vi "Parse Uplink.vi"(8 "error in (no error)":errorcluster, 10 "Uplink":u8[][](array[numeric]) format="%02x") -> (0 "error out":errorcluster, 1 "Data":string, 2 "Response Code":string, 3 "Response Token":string, 4 "tChecksum Valid":bool, 5 "CP_DATA":u8[](array[numeric]), 6 "bChecksum Valid":bool)   [LabVIEW 2009]
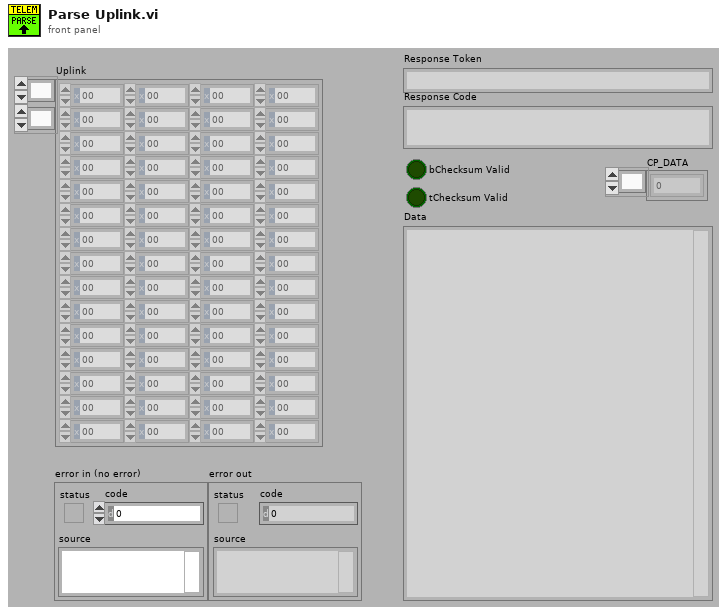
[diagram p1: front panel]
types:
  T1 = cluster{"FirstBlockFlag":u8, "respToken":u8, "cmdToken":u16, "cmdData":u8[], "b1ChkSum":u8, "tChkSum":u8, "tChkSumCalc":u8, "b1ChkSumCalc":u8}
  T2 = cluster{"Boolean array[0]":bool, "Boolean array[1]":bool, "Boolean array[2]":bool, "Boolean array[3]":bool, "Boolean array[4]":bool, "Boolean array[5]":bool, "Boolean array[6]":bool, "Boolean array[7]":bool}
  T3 = cluster{"Boolean array[0]":bool, "Boolean array[1]":bool, "Boolean array[2]":bool, "Boolean array[3]":bool, "Boolean array[4]":bool, "Boolean array[5]":bool, "Boolean array[6]":bool, "Boolean array[7]":bool, "Boolean array[8]":bool, "Boolean array[9]":bool, "Boolean array[10]":bool, "Boolean array[11]":bool, "Boolean array[12]":bool, "Boolean array[13]":bool, "Boolean array[14]":bool, "Boolean array[15]":bool}
  T4 = cluster{"DATA[0]":u8, "DATA[1]":u8, "DATA[2]":u8, "DATA[3]":u8, "DATA[4]":u8, "DATA[5]":u8, "DATA[6]":u8, "DATA[7]":u8}
  T5 = cluster{"[0]":string, "[1]":string, "[2]":string, "[3]":string, "[4]":string, "[5]":string, "[6]":string, "[7]":string, "[8]":string, "[9]":string}
  T6 = cluster{"DATA[0]":u8, "DATA[1]":u8, "DATA[2]":u8, "DATA[3]":u8, "DATA[4]":u8, "DATA[5]":u8, "DATA[6]":u8, "DATA[7]":u8, "DATA[8]":u8, "DATA[9]":u8, "DATA[10]":u8, "DATA[11]":u8, "DATA[12]":u8, "DATA[13]":u8, "DATA[14]":u8, "DATA[15]":u8}
  T7 = cluster{"[0]":u8, "[1]":u8, "[2]":u8, "[3]":u8, "[4]":u8, "[5]":u8, "[6]":u8, "[7]":u8, "[8]":u8, "[9]":u8, "[10]":u8, "[11]":u8, "[12]":u8, "[13]":u8, "[14]":u8, "[15]":u8, "[16]":u8, "[17]":u8, "[18]":u8, "[19]":u8, "[20]":u8, "[21]":u8, "[22]":u8, "[23]":u8, "[24]":u8, "[25]":u8, "[26]":u8, "[27]":u8, "[28]":u8, "[29]":u8, "[30]":u8, "[31]":u8, "[32]":u8, "[33]":u8, "[34]":u8, "[35]":u8, "[36]":u8, "[37]":u8, "[38]":u8, "[39]":u8, "[40]":u8, "[41]":u8, "[42]":u8, "[43]":u8, "[44]":u8, "[45]":u8, "[46]":u8, "[47]":u8, "[48]":u8, "[49]":u8, "[50]":u8, "[51]":u8, "[52]":u8, "[53]":u8}
  T8 = cluster{"DATA[0]":u8, "DATA[1]":u8, "DATA[2]":u8, "DATA[3]":u8, "DATA[4]":u8, "DATA[5]":u8, "DATA[6]":u8, "DATA[7]":u8, "DATA[8]":u8, "DATA[9]":u8, "DATA[10]":u8, "DATA[11]":u8, "DATA[12]":u8, "DATA[13]":u8, "DATA[14]":u8, "DATA[15]":u8, "DATA[16]":u8, "DATA[17]":u8, "DATA[18]":u8, "DATA[19]":u8, "DATA[20]":u8, "DATA[21]":u8, "DATA[22]":u8, "DATA[23]":u8, "DATA[24]":u8, "DATA[25]":u8, "DATA[26]":u8, "DATA[27]":u8, "DATA[28]":u8, "DATA[29]":u8, "DATA[30]":u8, "DATA[31]":u8, "DATA[32]":u8, "DATA[33]":u8, "DATA[34]":u8, "DATA[35]":u8, "DATA[36]":u8, "DATA[37]":u8, "DATA[38]":u8, "DATA[39]":u8, "DATA[40]":u8, "DATA[41]":u8, "DATA[42]":u8, "DATA[43]":u8, "DATA[44]":u8, "DATA[45]":u8, "DATA[46]":u8}
  T9 = cluster{"DATA[0]":u8, "DATA[1]":u8, "DATA[2]":u8, "DATA[3]":u8, "DATA[4]":u8, "DATA[5]":u8, "DATA[6]":u8, "DATA[7]":u8, "DATA[8]":u8, "DATA[9]":u8, "DATA[10]":u8, "DATA[11]":u8, "DATA[12]":u8, "DATA[13]":u8, "DATA[14]":u8, "DATA[15]":u8, "DATA[16]":u8, "DATA[17]":u8, "DATA[18]":u8, "DATA[19]":u8, "DATA[20]":u8, "DATA[21]":u8, "DATA[22]":u8, "DATA[23]":u8}
  T10 = cluster{"Boolean array[0]":bool, "Boolean array[1]":bool, "Boolean array[2]":bool, "Boolean array[3]":bool, "Boolean array[4]":bool, "Boolean array[5]":bool, "Boolean array[6]":bool, "Boolean array[7]":bool, "Boolean array[8]":bool}
  T11 = cluster{"[0]":u8, "[1]":u8, "[2]":u8, "[3]":u8, "[4]":u8, "[5]":u8, "[6]":u8, "[7]":u8}
  T12 = cluster{"[0]":u8, "[1]":u8, "[2]":u8, "[3]":u8, "[4]":u8, "[5]":u8, "[6]":u8, "[7]":u8, "[8]":u8, "[9]":u8, "[10]":u8, "[11]":u8, "[12]":u8, "[13]":u8, "[14]":u8, "[15]":u8, "[16]":u8, "[17]":u8, "[18]":u8, "[19]":u8, "[20]":u8, "[21]":u8, "[22]":u8, "[23]":u8, "[24]":u8, "[25]":u8, "[26]":u8, "[27]":u8, "[28]":u8, "[29]":u8, "[30]":u8, "[31]":u8, "[32]":u8, "[33]":u8, "[34]":u8, "[35]":u8, "[36]":u8, "[37]":u8}
  T13 = cluster{"[0]":u8, "[1]":u8, "[2]":u8, "[3]":u8, "[4]":u8, "[5]":u8}
  T14 = cluster{"DATA[0]":u8, "DATA[1]":u8, "DATA[2]":u8, "DATA[3]":u8, "DATA[4]":u8, "DATA[5]":u8}
  T15 = cluster{"DATA[0]":u8, "DATA[1]":u8, "DATA[2]":u8, "DATA[3]":u8, "DATA[4]":u8, "DATA[5]":u8, "DATA[6]":u8, "DATA[7]":u8, "DATA[8]":u8, "DATA[9]":u8, "DATA[10]":u8, "DATA[11]":u8, "DATA[12]":u8, "DATA[13]":u8, "DATA[14]":u8, "DATA[15]":u8, "DATA[16]":u8}
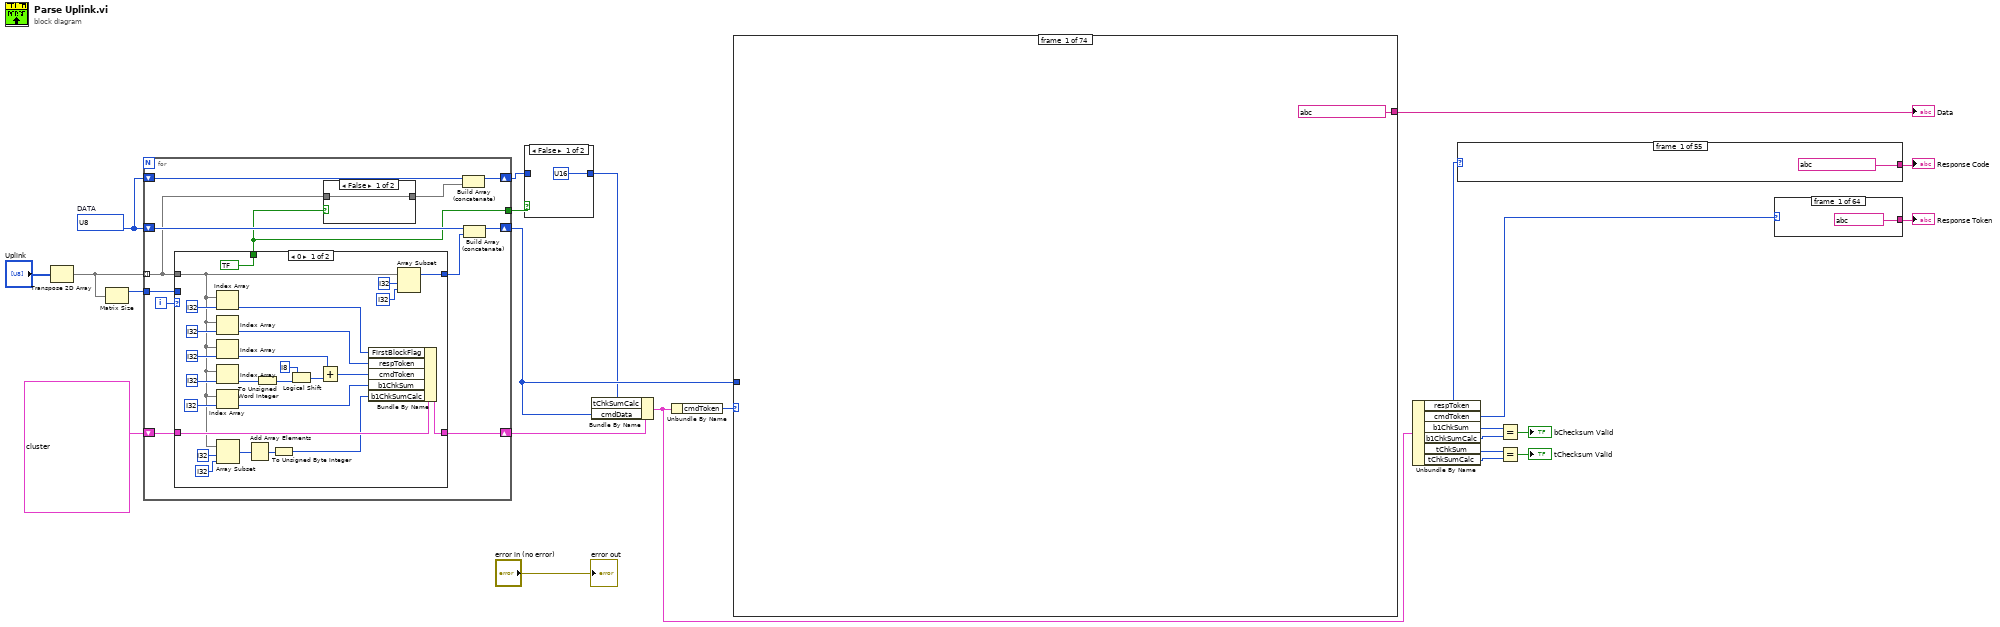
[diagram p0: block diagram]
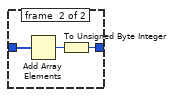
[diagram p2: hidden frame]
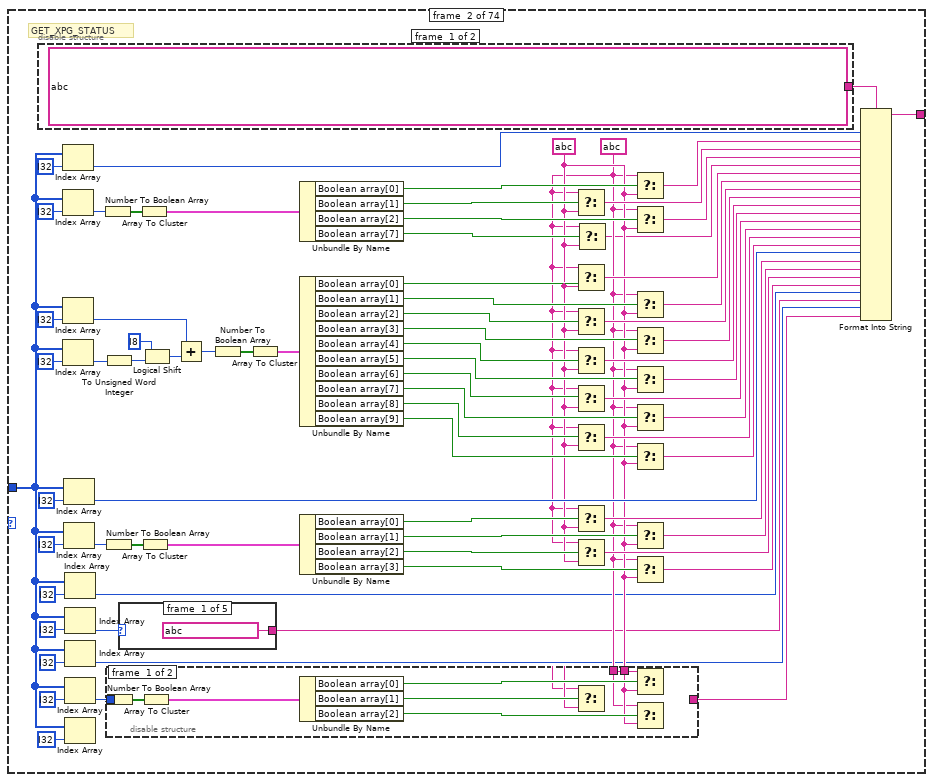
[diagram p3: hidden frame]
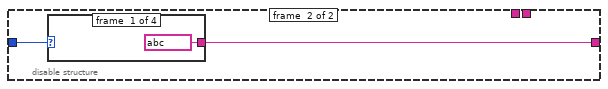
[diagram p4: hidden frame]
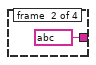
[diagram p5: hidden frame]
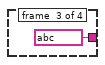
[diagram p6: hidden frame]
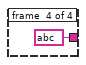
[diagram p7: hidden frame]
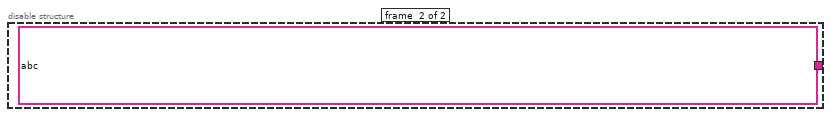
[diagram p8: hidden frame]
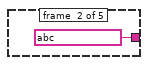
[diagram p9: hidden frame]
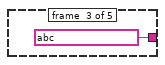
[diagram p10: hidden frame]
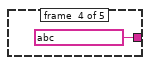
[diagram p11: hidden frame]
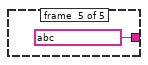
[diagram p12: hidden frame]
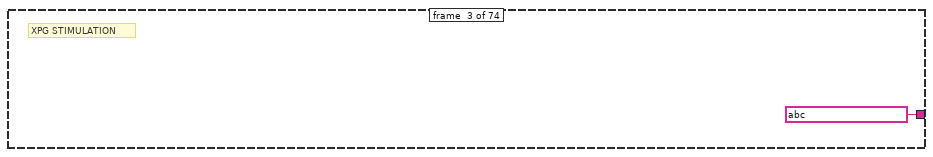
[diagram p13: hidden frame]
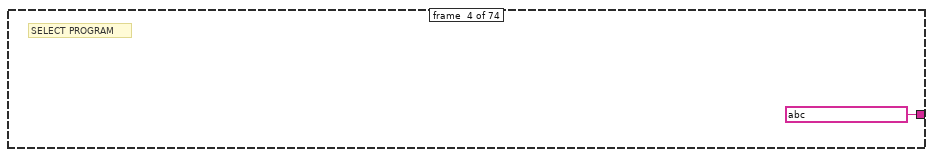
[diagram p14: hidden frame]
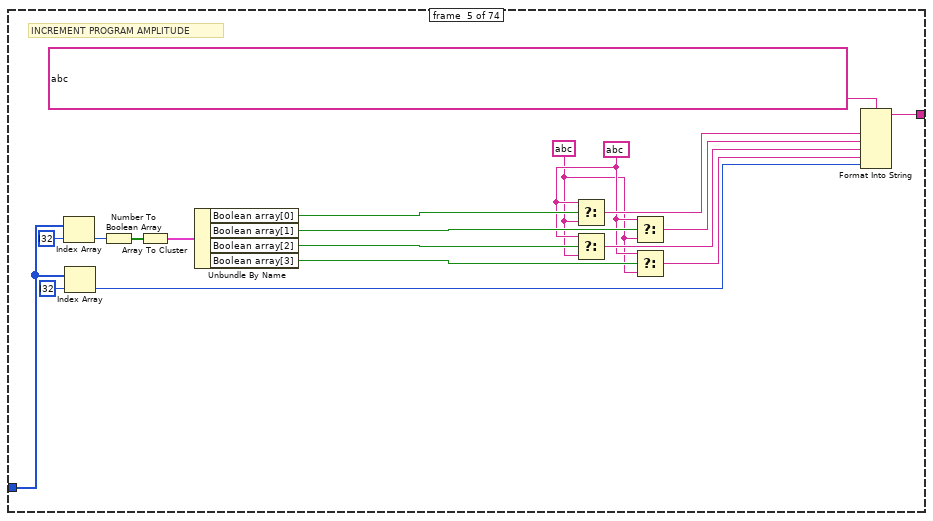
[diagram p15: hidden frame]
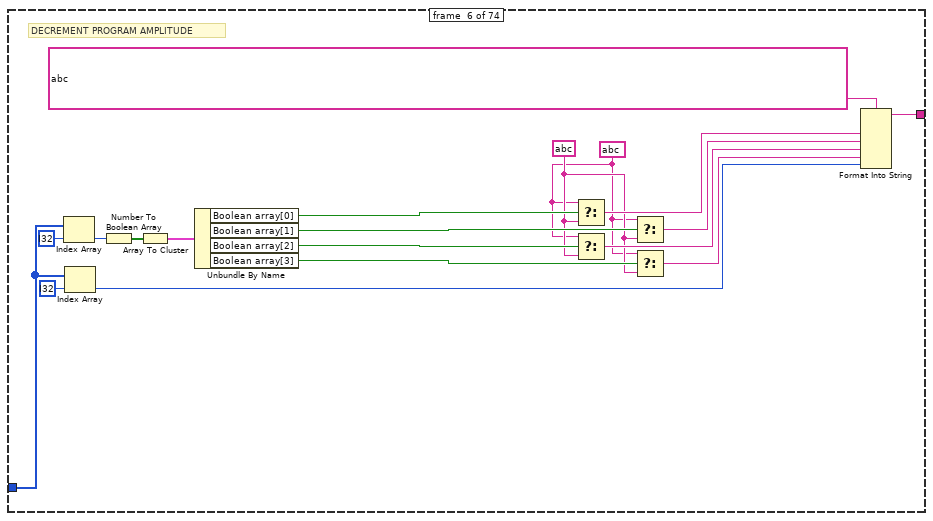
[diagram p16: hidden frame]
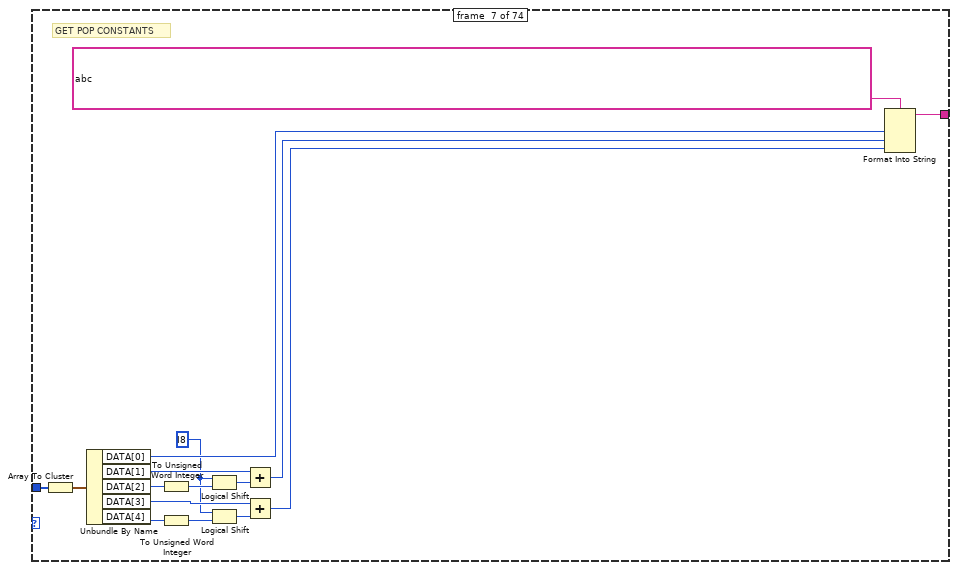
[diagram p17: hidden frame]
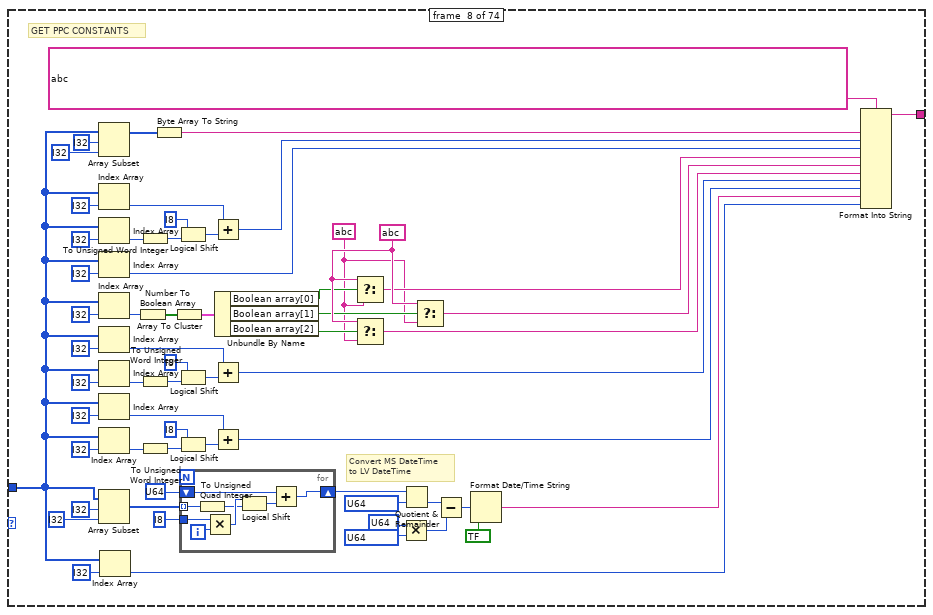
[diagram p18: hidden frame]
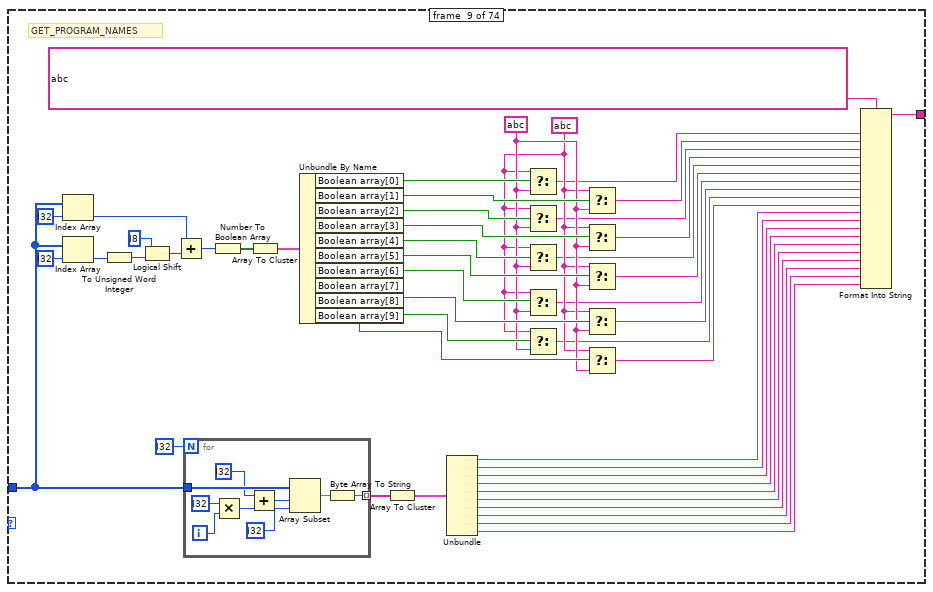
[diagram p19: hidden frame]
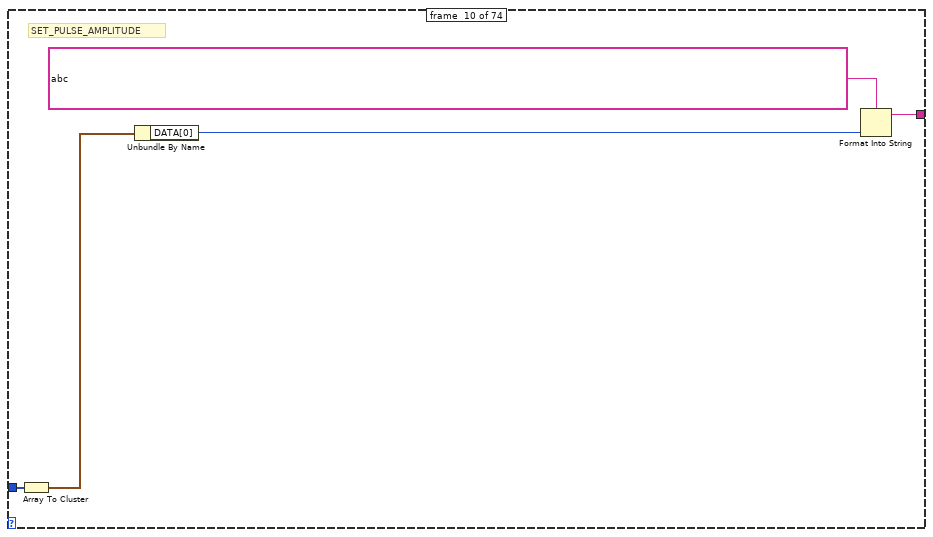
[diagram p20: hidden frame]
diagram:
  w13 = u8[] ?  # DATA
  n1 = Transpose 2D Array(2D array="Uplink") -> (transposed array=w15:u8[][])
  n2 = Matrix Size(0:w15) -> (1:w21:i32)  [unwired: 1 out]
  n3 = for {
    tunnel: w15 -> [w27] mode=indexing
    shift-right: [w31] -> w19
    shift-left: w13 -> [w32]
    shift-right: [w34] -> w20
    shift-left: T1 ? -> [w35]
    tunnel: w21 -> [w33]
    shift-right: [w28] -> w12
    shift-left: w13 -> [w29]
    tunnel: [w25] -> w11
    i -> [w36]
    n4 = case shown="0" w36 {
      selector: w36 -> [_ w79]
      tunnel: w27 -> [w45 w69]
      tunnel: [w65 w75] -> w30
      tunnel: w35 -> [w59 w70]
      tunnel: [w58 w71] -> w34
      tunnel: w33 -> [_ w77]
      tunnel: [bool ? w68] -> w25
      frame #0 {
        n5 = Index Array(array=w45, index=i32 ?) -> (element=w57:u8)
        n6 = Index Array(array=w45, index=i32 ?) -> (element=w54:u8)
        n7 = Index Array(array=w45, index=i32 ?) -> (element=w49:u8)
        n8 = Index Array(array=w45, index=i32 ?) -> (element=w53:u8)
        n9 = Index Array(array=w45, index=i32 ?) -> (element=w56:u8)
        n10 = Array Subset(array=w45, index=i32 ?, length=i32 ?) -> (w42:u8[])
        n11 = Add Array Elements(numeric array=w42) -> (sum=w44:u8)
        n12 = To Unsigned Word Integer(number=w53) -> (unsigned 16bit integer=w55:u16)
        n13 = To Unsigned Byte Integer(number=w44) -> (unsigned 8bit integer=w43:u8)
        n14 = Logical Shift(y=i8 ?, x=w55) -> (x << y=w51:u16)
        n15 = Add(x=w49, y=w51) -> (x+y=w50:u16)
        n16 = Bundle By Name(cluster=w59, "FirstBlockFlag"=w57, "respToken"=w54, "cmdToken"=w50, "b1ChkSum"=w56, "b1ChkSumCalc"=w43) -> (w58:T1)
        n17 = Array Subset(array=w45, index=i32 ?, length=i32 ?) -> (w65:u8[])
      }
      frame #1 {
        # "If Last Packet of Multi-Packet\nUplink, truncate Data Read\nand store tChkSum"
        n18 = Increment(x=w79) -> (x+1=w78:i32)
        n19 = Equal?(x=w77, y=w78) -> (x = y?=w68:bool)
        n20 = case shown="True" w68 {
          tunnel: [w80 w84] -> w71
          tunnel: w70 -> [w80 w85]
          tunnel: w69 -> [_ w82]
          frame #0 {
          }
          frame #1 {
            n21 = Index Array(array=w82, index=i32 ?) -> (element=w83:u8)
            n22 = Bundle By Name(cluster=w85, "tChkSum"=w83) -> (w84:T1)
          }
        }
        n23 = Select(t=i32 ? ("length"), s=w68, f=i32 ? ("length")) -> (s? t:f=w74:i32)
        n24 = Array Subset(array=w69, index=i32 ?, length=w74) -> (w75:u8[])
      }
    }
    n25 = case shown="False" w25 {
      tunnel: w27 -> [w37 w40]
      tunnel: [w37 w39] -> w26
      frame #0 {
      }
      frame #1 {
        n26 = Array Subset(array=w40, index=i32 ?, length=i32 ?) -> (w39:u8[])
      }
    }
    n27 = Build Array (concatenate)(w29, w26) -> (w28:u8[])
    n28 = Build Array (concatenate)(w32, w30) -> (w31:u8[])
  }
  n29 = case shown="False" w11 {
    tunnel: w12 -> [_ w87]
    tunnel: [u16 ? ("CRC16r") w88] -> w2
    frame #0 {
    }
    frame #1 {
      n30 = Add Array Elements(numeric array=w87) -> (sum=w89:u8)
      n31 = To Unsigned Byte Integer(number=w89) -> (unsigned 8bit integer=w88:u8)
    }
  }
  n32 = Bundle By Name(cluster=w20, "tChkSumCalc"=w2, "cmdData"=w19) -> (w4:T1)
  n33 = Unbundle By Name(w4) -> ("cmdToken"=w1:u16)
  n34 = case shown="3" w1 {
    tunnel: w19 -> [_ w100 _ _ w194 w213 w232 w241 w323 w369 w374 w379 w395 _ w414 w419 w424 _ w430 w435 w450 w469 _ _ w478 _ w615 _ w648 _ w798 _ w807 _ w855 _ w902 _ w928 _ w954 w962 w998 w1020 _ w1028 _ w1053 w1058 w1073 _ w1166 _ w1191 _ w1200 _ w1260 _ w1316 _ w1321 _ _ _ w1335 _ _ _ _ w1363 _ w1431 _]
    tunnel: [string ? w162 string ? string ? w204 w223 w239 w300 w356 w370 w375 w380 w409 string ? w415 w420 w425 string ? w431 w436 w451 w473 string ? string ? w517 string ? w626 string ? w713 string ? w802 string ? w812 string ? w860 string ? w905 string ? w931 string ? w956 w973 w1000 w1022 string ? w1033 string ? w1055 w1062 w1104 string ? w1169 string ? w1196 string ? w1208 string ? w1267 string ? w1317 string ? w1329 _ _ string ? w1343 _ _ _ _ w1366 string ? w1433 string ?] -> w18
    frame #0 {
    }
    frame #1 {
      w98 = string ?
      w97 = string ?
      # "GET_XPG_STATUS"
      n35 = disable-structure shown="Enabled" {
        disable-tunnel: [_ string ? ("format string")] -> w91
        frame #0 {
          (unwired) string ? ("format string")
        }
        frame #1 {
        }
      }
      n36 = Index Array(array=w100, index=i32 ?) -> (element=w163:u8)
      n37 = Index Array(array=w100, index=i32 ?) -> (element=w147:u8)
      n38 = Index Array(array=w100, index=i32 ?) -> (element=w135:u8)
      n39 = Index Array(array=w100, index=i32 ?) -> (element=w136:u8)
      n40 = Index Array(array=w100, index=i32 ?) -> (element=w120:u8)
      n41 = Index Array(array=w100, index=i32 ?) -> (element=w118:u8)
      n42 = Index Array(array=w100, index=i32 ?) -> (element=w95:u8)
      n43 = Index Array(array=w100, index=i32 ?) -> (element=w105:u8)
      n44 = Index Array(array=w100, index=i32 ?) -> (element=w93:u8)
      n45 = Index Array(array=w100, index=i32 ?) -> (element=w102:u8)
      n46 = Index Array(array=w100, index=i32 ?) -> ()  [unwired: 1 out]
      n47 = Number To Boolean Array(number=w147) -> (Boolean array=w146:bool[])
      n48 = To Unsigned Word Integer(number=w136) -> (unsigned 16bit integer=w139:u16)
      n49 = Number To Boolean Array(number=w118) -> (Boolean array=w117:bool[])
      n50 = disable-structure shown="Enabled" {
        disable-tunnel: w102 -> [w172 w174]
        disable-tunnel: w98 -> [w166 _]
        disable-tunnel: w97 -> [w165 _]
        disable-tunnel: [_ w173] -> w92
        frame #0 {
          n51 = Number To Boolean Array(number=w172) -> (Boolean array=w171:bool[])
          n52 = Array To Cluster(array=w171) -> (cluster=w170:T2)
          n53 = Unbundle By Name(w170) -> ("Boolean array[0]"=w169:bool, "Boolean array[1]"=w168:bool, "Boolean array[2]"=w167:bool)
          n54 = Select(t=w165, s=w168, f=w166) -> ()  [unwired: 1 out]
          n55 = Select(t=w165, s=w169, f=w166) -> ()  [unwired: 1 out]
          n56 = Select(t=w165, s=w167, f=w166) -> ()  [unwired: 1 out]
        }
        frame #1 {
          n57 = case shown="3" w174 {
            tunnel: [string ? string ? string ? string ?] -> w173
            frame #0 {
            }
            frame #1 {
            }
            frame #2 {
            }
            frame #3 {
            }
          }
        }
      }
      n58 = case shown="4" w105 {
        tunnel: [string ? string ? string ? string ? string ?] -> w94
        frame #0 {
        }
        frame #1 {
        }
        frame #2 {
        }
        frame #3 {
        }
        frame #4 {
        }
      }
      n59 = Array To Cluster(array=w146) -> (cluster=w145:T2)
      n60 = Array To Cluster(array=w117) -> (cluster=w116:T2)
      n61 = Logical Shift(y=i8 ?, x=w139) -> (x << y=w137:u16)
      n62 = Add(x=w135, y=w137) -> (x+y=w133:u16)
      n63 = Number To Boolean Array(number=w133) -> (Boolean array=w134:bool[])
      n64 = Array To Cluster(array=w134) -> (cluster=w132:T3)
      n65 = Unbundle By Name(w145) -> ("Boolean array[0]"=w144:bool, "Boolean array[1]"=w143:bool, "Boolean array[2]"=w142:bool, "Boolean array[7]"=w99:bool)
      n66 = Unbundle By Name(w132) -> ("Boolean array[0]"=w131:bool, "Boolean array[1]"=w130:bool, "Boolean array[2]"=w129:bool, "Boolean array[3]"=w128:bool, "Boolean array[4]"=w127:bool, "Boolean array[5]"=w126:bool, "Boolean array[6]"=w125:bool, "Boolean array[7]"=w124:bool, "Boolean array[8]"=w123:bool, "Boolean array[9]"=w122:bool)
      n67 = Unbundle By Name(w116) -> ("Boolean array[0]"=w115:bool, "Boolean array[1]"=w114:bool, "Boolean array[2]"=w113:bool, "Boolean array[3]"=w112:bool)
      n68 = Select(t=w97, s=w143, f=w98) -> (s? t:f=w160:string)
      n69 = Select(t=w97, s=w131, f=w98) -> (s? t:f=w158:string)
      n70 = Select(t=w97, s=w129, f=w98) -> (s? t:f=w156:string)
      n71 = Select(t=w97, s=w127, f=w98) -> (s? t:f=w154:string)
      n72 = Select(t=w97, s=w125, f=w98) -> (s? t:f=w152:string)
      n73 = Select(t=w97, s=w123, f=w98) -> (s? t:f=w150:string)
      n74 = Select(t=w97, s=w115, f=w98) -> (s? t:f=w111:string)
      n75 = Select(t=w97, s=w113, f=w98) -> (s? t:f=w109:string)
      n76 = Select(t=w97, s=w99, f=w98) -> (s? t:f=w96:string)
      n77 = Select(t=w97, s=w144, f=w98) -> (s? t:f=w161:string)
      n78 = Select(t=w97, s=w142, f=w98) -> (s? t:f=w159:string)
      n79 = Select(t=w97, s=w130, f=w98) -> (s? t:f=w157:string)
      n80 = Select(t=w97, s=w128, f=w98) -> (s? t:f=w155:string)
      n81 = Select(t=w97, s=w126, f=w98) -> (s? t:f=w153:string)
      n82 = Select(t=w97, s=w124, f=w98) -> (s? t:f=w151:string)
      n83 = Select(t=w97, s=w122, f=w98) -> (s? t:f=w149:string)
      n84 = Select(t=w97, s=w114, f=w98) -> (s? t:f=w110:string)
      n85 = Select(t=w97, s=w112, f=w98) -> (s? t:f=w108:string)
      n86 = Format Into String(format string=w91, w163, w161, w160, w159, w96, w158, w157, w156, w155, w154, w153, w152, w151, w150, w149, w120, w111, w110, w109, w108, w95, w94, w93, w92) -> (resulting string=w162:string)  [unwired: 2 in, 1 out]
    }
    frame #2 {
      # "XPG STIMULATION"
    }
    frame #3 {
      # "SELECT PROGRAM"
    }
    frame #4 {
      w187 = string ?
      w188 = string ?
      # "INCREMENT PROGRAM AMPLITUDE"
      n87 = Index Array(array=w194, index=i32 ?) -> (element=w202:u8)
      n88 = Index Array(array=w194, index=i32 ?) -> (element=w189:u8)
      n89 = Number To Boolean Array(number=w202) -> (Boolean array=w201:bool[])
      n90 = Array To Cluster(array=w201) -> (cluster=w200:T2)
      n91 = Unbundle By Name(w200) -> ("Boolean array[0]"=w199:bool, "Boolean array[1]"=w198:bool, "Boolean array[2]"=w197:bool, "Boolean array[3]"=w196:bool)
      n92 = Select(t=w188, s=w199, f=w187) -> (s? t:f=w193:string)
      n93 = Select(t=w188, s=w197, f=w187) -> (s? t:f=w191:string)
      n94 = Select(t=w188, s=w198, f=w187) -> (s? t:f=w192:string)
      n95 = Select(t=w188, s=w196, f=w187) -> (s? t:f=w190:string)
      n96 = Format Into String(format string=string ?, w193, w192, w191, w190, w189) -> (resulting string=w204:string)  [unwired: 2 in, 1 out]
    }
    frame #5 {
      w207 = string ?
      w206 = string ?
      # "DECREMENT PROGRAM AMPLITUDE"
      n97 = Index Array(array=w213, index=i32 ?) -> (element=w221:u8)
      n98 = Index Array(array=w213, index=i32 ?) -> (element=w208:u8)
      n99 = Number To Boolean Array(number=w221) -> (Boolean array=w220:bool[])
      n100 = Array To Cluster(array=w220) -> (cluster=w219:T2)
      n101 = Unbundle By Name(w219) -> ("Boolean array[0]"=w218:bool, "Boolean array[1]"=w217:bool, "Boolean array[2]"=w216:bool, "Boolean array[3]"=w215:bool)
      n102 = Select(t=w206, s=w218, f=w207) -> (s? t:f=w212:string)
      n103 = Select(t=w206, s=w216, f=w207) -> (s? t:f=w210:string)
      n104 = Select(t=w206, s=w217, f=w207) -> (s? t:f=w211:string)
      n105 = Select(t=w206, s=w215, f=w207) -> (s? t:f=w209:string)
      n106 = Format Into String(format string=string ?, w212, w211, w210, w209, w208) -> (resulting string=w223:string)  [unwired: 2 in, 1 out]
    }
    frame #6 {
      w225 = i8 ? ("y")
      # "GET POP CONSTANTS"
      n107 = Array To Cluster(array=w232) -> (cluster=w231:T4)
      n108 = Unbundle By Name(w231) -> ("DATA[0]"=w230:u8, "DATA[1]"=w229:u8, "DATA[2]"=w228:u8, "DATA[3]"=w227:u8, "DATA[4]"=w226:u8)
      n109 = To Unsigned Word Integer(number=w228) -> (unsigned 16bit integer=w238:u16)
      n110 = To Unsigned Word Integer(number=w226) -> (unsigned 16bit integer=w236:u16)
      n111 = Logical Shift(y=w225, x=w238) -> (x << y=w237:u16)
      n112 = Logical Shift(y=w225, x=w236) -> (x << y=w235:u16)
      n113 = Add(x=w229, y=w237) -> (x+y=w234:u16)
      n114 = Add(x=w227, y=w235) -> (x+y=w233:u16)
      n115 = Format Into String(format string=string ?, w230, w234, w233) -> (resulting string=w239:string)  [unwired: 2 in, 1 out]
    }
    frame #7 {
      w243 = string ?
      w281 = string ?
      # "Convert MS DateTime\nto LV DateTime"
      # "GET PPC CONSTANTS"
      n116 = Array Subset(array=w241, index=i32 ?, length=i32 ?) -> (w297:u8[])
      n117 = Index Array(array=w241, index=i32 ?) -> (element=w289:u8)
      n118 = Index Array(array=w241, index=i32 ?) -> (element=w290:u8)
      n119 = Index Array(array=w241, index=i32 ?) -> (element=w286:u8)
      n120 = Index Array(array=w241, index=i32 ?) -> (element=w284:u8)
      n121 = Index Array(array=w241, index=i32 ?) -> (element=w268:u8)
      n122 = Index Array(array=w241, index=i32 ?) -> (element=w269:u8)
      n123 = Index Array(array=w241, index=i32 ?) -> (element=w260:u8)
      n124 = Index Array(array=w241, index=i32 ?) -> (element=w261:u8)
      n125 = Array Subset(array=w241, index=i32 ?, length=i32 ?) -> (w256:u8[])
      n126 = Index Array(array=w241, index=i32 ?) -> (element=w246:u8)
      n127 = Number To Boolean Array(number=w284) -> (Boolean array=w283:bool[])
      n128 = To Unsigned Word Integer(number=w290) -> (unsigned 16bit integer=w293:u16)
      n129 = To Unsigned Word Integer(number=w269) -> (unsigned 16bit integer=w272:u16)
      n130 = To Unsigned Word Integer(number=w261) -> (unsigned 16bit integer=w264:u16)
      n131 = Byte Array To String(unsigned byte array=w297) -> (string=w296:string)
      n132 = Array To Cluster(array=w283) -> (cluster=w282:T2)
      n133 = Logical Shift(y=i8 ?, x=w293) -> (x << y=w291:u16)
      n134 = Logical Shift(y=i8 ?, x=w272) -> (x << y=w270:u16)
      n135 = Logical Shift(y=i8 ?, x=w264) -> (x << y=w262:u16)
      n136 = for {
        tunnel: w256 -> [w309] mode=indexing
        shift-right: [w303] -> w251
        shift-left: u64 ? ("y") -> [w304]
        tunnel: i8 ? ("y") -> [w307]
        i -> [w308]
        n137 = To Unsigned Quad Integer(1:w309) -> (0:w302:u64)
        n138 = Multiply(x=w307, y=w308) -> (x*y=w306:i32)
        n139 = Logical Shift(y=w306, x=w302) -> (x << y=w305:u64)
        n140 = Add(x=w304, y=w305) -> (x+y=w303:u64)
      }
      n141 = Add(x=w289, y=w291) -> (x+y=w288:u16)
      n142 = Add(x=w268, y=w270) -> (x+y=w267:u16)
      n143 = Add(x=w260, y=w262) -> (x+y=w259:u16)
      n144 = Unbundle By Name(w282) -> ("Boolean array[0]"=w279:bool, "Boolean array[1]"=w280:bool, "Boolean array[2]"=w278:bool)
      n145 = Select(t=w281, s=w279, f=w243) -> (s? t:f=w277:string)
      n146 = Select(t=w281, s=w278, f=w243) -> (s? t:f=w275:string)
      n147 = Multiply(x=u64 ? ("y"), y=u64 ?) -> (x*y=w249:u64)
      n148 = Quotient & Remainder(x=w251, y=u64 ?) -> (floor(x/y)=w242:u64)  [unwired: 1 out]
      n149 = Select(t=w281, s=w280, f=w243) -> (s? t:f=w276:string)
      n150 = Subtract(x=w242, y=w249) -> (x-y=w245:u64)
      n151 = Format Date/Time String(seconds (now)=w245, UTC format=bool ?) -> (date/time string=w244:string)  [unwired: 1 in]
      n152 = Format Into String(format string=string ?, w296, w288, w286, w277, w276, w275, w267, w259, w244, w246) -> (resulting string=w300:string)  [unwired: 2 in, 1 out]
    }
    frame #8 {
      w335 = string ?
      w334 = string ?
      # "GET_PROGRAM_NAMES"
      n153 = Index Array(array=w323, index=i32 ?) -> (element=w349:u8)
      n154 = Index Array(array=w323, index=i32 ?) -> (element=w350:u8)
      n155 = To Unsigned Word Integer(number=w350) -> (unsigned 16bit integer=w353:u16)
      n156 = Logical Shift(y=i8 ?, x=w353) -> (x << y=w351:u16)
      n157 = Add(x=w349, y=w351) -> (x+y=w347:u16)
      n158 = for {
        N: i32 ? -> [_]
        tunnel: w323 -> [w366]
        tunnel: [w358] -> w322 mode=indexing
        i -> [w364]
        n159 = Multiply(x=i32 ?, y=w364) -> (x*y=w362:i32)
        n160 = Add(x=i32 ?, y=w362) -> (x+y=w360:i32)
        n161 = Array Subset(array=w366, index=w360, length=i32 ?) -> (w359:u8[])
        n162 = Byte Array To String(unsigned byte array=w359) -> (string=w358:string)
      }
      n163 = Number To Boolean Array(number=w347) -> (Boolean array=w348:bool[])
      n164 = Array To Cluster(array=w348) -> (cluster=w346:T3)
      n165 = Unbundle By Name(w346) -> ("Boolean array[0]"=w345:bool, "Boolean array[1]"=w344:bool, "Boolean array[2]"=w343:bool, "Boolean array[3]"=w342:bool, "Boolean array[4]"=w341:bool, "Boolean array[5]"=w340:bool, "Boolean array[6]"=w339:bool, "Boolean array[7]"=w338:bool, "Boolean array[8]"=w337:bool, "Boolean array[9]"=w336:bool)
      n166 = Array To Cluster(array=w322) -> (cluster=w321:T5)
      n167 = Unbundle(w321) -> ("[0]"=w319:string, "[1]"=w318:string, "[2]"=w317:string, "[3]"=w316:string, "[4]"=w315:string, "[5]"=w314:string, "[6]"=w313:string, "[7]"=w312:string, "[8]"=w311:string, "[9]"=w310:string)
      n168 = Select(t=w334, s=w345, f=w335) -> (s? t:f=w333:string)
      n169 = Select(t=w334, s=w343, f=w335) -> (s? t:f=w331:string)
      n170 = Select(t=w334, s=w341, f=w335) -> (s? t:f=w329:string)
      n171 = Select(t=w334, s=w339, f=w335) -> (s? t:f=w327:string)
      n172 = Select(t=w334, s=w337, f=w335) -> (s? t:f=w325:string)
      n173 = Select(t=w334, s=w344, f=w335) -> (s? t:f=w332:string)
      n174 = Select(t=w334, s=w342, f=w335) -> (s? t:f=w330:string)
      n175 = Select(t=w334, s=w340, f=w335) -> (s? t:f=w328:string)
      n176 = Select(t=w334, s=w338, f=w335) -> (s? t:f=w326:string)
      n177 = Select(t=w334, s=w336, f=w335) -> (s? t:f=w324:string)
      n178 = Format Into String(format string=string ?, w333, w332, w331, w330, w329, w328, w327, w326, w325, w324, w319, w318, w317, w316, w315, w314, w313, w312, w311, w310) -> (resulting string=w356:string)  [unwired: 2 in, 1 out]
    }
    frame #9 {
      # "SET_PULSE_AMPLITUDE"
      n179 = Array To Cluster(array=w369) -> (cluster=w368:T4)
      n180 = Unbundle By Name(w368) -> ("DATA[0]"=w367:u8)
      n181 = Format Into String(format string=string ?, w367) -> (resulting string=w370:string)  [unwired: 2 in, 1 out]
    }
    frame #10 {
      # "INCREMENT_PULSE_AMPLITUDE"
      n182 = Array To Cluster(array=w374) -> (cluster=w373:T4)
      n183 = Unbundle By Name(w373) -> ("DATA[0]"=w372:u8)
      n184 = Format Into String(format string=string ?, w372) -> (resulting string=w375:string)  [unwired: 2 in, 1 out]
    }
    frame #11 {
      # "DECREMENT_PULSE_AMPLITUDE"
      n185 = Array To Cluster(array=w379) -> (cluster=w378:T4)
      n186 = Unbundle By Name(w378) -> ("DATA[0]"=w377:u8)
      n187 = Format Into String(format string=string ?, w377) -> (resulting string=w380:string)  [unwired: 2 in, 1 out]
    }
    frame #12 {
      w397 = string ?
      w398 = string ?
      # "GET_PULSE_WIDTHS"
      n188 = Array To Cluster(array=w395) -> (cluster=w396:T6)
      n189 = Unbundle By Name(w396) -> ("DATA[0]"=w394:u8, "DATA[3]"=w383:u8, "DATA[2]"=w382:u8, "DATA[5]"=w385:u8, "DATA[4]"=w384:u8, "DATA[7]"=w387:u8, "DATA[6]"=w386:u8, "DATA[9]"=w389:u8, "DATA[8]"=w388:u8)
      n190 = Join Numbers(hi=w383, lo=w382) -> ((hi.lo)=w393:u16)
      n191 = Join Numbers(hi=w385, lo=w384) -> ((hi.lo)=w392:u16)
      n192 = Join Numbers(hi=w387, lo=w386) -> ((hi.lo)=w391:u16)
      n193 = Join Numbers(hi=w389, lo=w388) -> ((hi.lo)=w390:u16)
      n194 = Number To Boolean Array(number=w394) -> (Boolean array=w408:bool[])
      n195 = Array To Cluster(array=w408) -> (cluster=w407:T2)
      n196 = Unbundle By Name(w407) -> ("Boolean array[0]"=w406:bool, "Boolean array[1]"=w405:bool, "Boolean array[2]"=w404:bool, "Boolean array[3]"=w403:bool)
      n197 = Select(t=w398, s=w406, f=w397) -> (s? t:f=w402:string)
      n198 = Select(t=w398, s=w404, f=w397) -> (s? t:f=w400:string)
      n199 = Select(t=w398, s=w405, f=w397) -> (s? t:f=w401:string)
      n200 = Select(t=w398, s=w403, f=w397) -> (s? t:f=w399:string)
      n201 = Format Into String(format string=string ?, w402, w401, w400, w399, w393, w392, w391, w390) -> (resulting string=w409:string)  [unwired: 2 in, 1 out]
    }
    frame #13 {
      # "SET_PULSE_WIDTHS"
    }
    frame #14 {
      # "INCREMENT_PULSE_WIDTH"
      n202 = Array To Cluster(array=w414) -> (cluster=w413:T4)
      n203 = Unbundle By Name(w413) -> ("DATA[0]"=w412:u8)
      n204 = Format Into String(format string=string ?, w412) -> (resulting string=w415:string)  [unwired: 2 in, 1 out]
    }
    frame #15 {
      # "DECREMENT_PULSE_WIDTH"
      n205 = Array To Cluster(array=w419) -> (cluster=w418:T4)
      n206 = Unbundle By Name(w418) -> ("DATA[0]"=w417:u8)
      n207 = Format Into String(format string=string ?, w417) -> (resulting string=w420:string)  [unwired: 2 in, 1 out]
    }
    frame #16 {
      # "GET_PROGRAM_FREQUENCY"
      n208 = Array To Cluster(array=w424) -> (cluster=w423:T4)
      n209 = Unbundle By Name(w423) -> ("DATA[0]"=w422:u8)
      n210 = Format Into String(format string=string ?, w422) -> (resulting string=w425:string)  [unwired: 2 in, 1 out]
    }
    frame #17 {
      # "SET_PROGRAM_FREQUENCY"
    }
    frame #18 {
      # "INCREMENT_PROGRAM_FREQUENCY"
      n211 = Array To Cluster(array=w430) -> (cluster=w429:T4)
      n212 = Unbundle By Name(w429) -> ("DATA[0]"=w428:u8)
      n213 = Format Into String(format string=string ?, w428) -> (resulting string=w431:string)  [unwired: 2 in, 1 out]
    }
    frame #19 {
      # "DECREMENT_PROGRAM_FREQUENCY"
      n214 = Array To Cluster(array=w435) -> (cluster=w434:T4)
      n215 = Unbundle By Name(w434) -> ("DATA[0]"=w433:u8)
      n216 = Format Into String(format string=string ?, w433) -> (resulting string=w436:string)  [unwired: 2 in, 1 out]
    }
    frame #20 {
      # "CHARGING_CONTROL"
      n217 = Array To Cluster(array=w450) -> (cluster=w449:T4)
      n218 = Unbundle By Name(w449) -> ("DATA[0]"=w444:u8, "DATA[1]"=w438:u8)
      n219 = And(x=i32 ?, y=w444) -> (x .and. y?=w443:i32)
      n220 = And(x=i32 ?, y=w444) -> (x .and. y?=w446:i32)
      n221 = And(x=w444, y=u8 ?) -> (x .and. y?=w439:u8)
      n222 = Greater Than 0?(x=w443) -> (x > 0?=w442:bool)
      n223 = case shown="True" w442 {
        tunnel: [string ? string ?] -> w441
        frame #0 {
        }
        frame #1 {
        }
      }
      n224 = case shown="4" w446 {
        tunnel: [string ? string ? string ? string ? string ?] -> w440
        frame #0 {
        }
        frame #1 {
        }
        frame #2 {
        }
        frame #3 {
        }
        frame #4 {
        }
      }
      n225 = Format Into String(format string=string ?, w440, w441, w439, w438) -> (resulting string=w451:string)  [unwired: 2 in, 1 out]
    }
    frame #21 {
      # "GET_XPG_IDENTITY"
      n226 = Array Subset(array=w469, index=i32 ?, length=i32 ?) -> (w470:u8[])
      n227 = Array Subset(array=w469, index=i32 ? ("length"), length=i32 ?) -> (w471:u8[])
      n228 = Array Subset(array=w469, index=i32 ? ("length"), length=i32 ?) -> (w472:u8[])
      n229 = Byte Array To String(unsigned byte array=w470) -> (string=w462:string)
      n230 = Byte Array To String(unsigned byte array=w471) -> (string=w461:string)
      n231 = Byte Array To String(unsigned byte array=w472) -> (string=w460:string)
      n232 = Format Into String(format string=string ?, w462, w461, w460) -> (resulting string=w473:string)  [unwired: 2 in, 1 out]
    }
    frame #22 {
      # "SET_XPG_IDENTITY"
    }
    frame #23 {
      # "RESTORE_PROGRAM_DEFAULTS"
    }
    frame #24 {
      w492 = string ?
      w491 = string ?
      # "GET_PROGRAM_DEFINITION"
      n233 = Index Array(array=w478, index=i32 ?) -> (element=w479:u8)
      n234 = Index Array(array=w478, index=i32 ?) -> (element=w513:u8)
      n235 = Index Array(array=w478, index=i32 ?) -> (element=w511:u8)
      n236 = Index Array(array=w478, index=i32 ?) -> (element=w483:u8)
      n237 = Index Array(array=w478, index=i32 ?) -> (element=w489:u8)
      n238 = for {
        N: i32 ? -> [_]
        tunnel: w478 -> [w570]
        shift-right: [w564] -> w482
        shift-left: string ? -> [w565]
        i -> [w519]
        w529 = i32 ? ("index")
        w569 = i32 ? ("length")
        n239 = Multiply(x=w519, y=w569) -> (x*y=w567:i32)
        n240 = Add(x=i32 ? ("index"), y=w567) -> (x+y=w568:i32)
        n241 = Array Subset(array=w570, index=w568, length=w569) -> (w526:u8[])
        n242 = case shown="3" w519 {
          tunnel: [string ? ("format string") string ? ("format string") string ? ("format string") string ? ("format string")] -> w561
          frame #0 {
          }
          frame #1 {
          }
          frame #2 {
          }
          frame #3 {
          }
        }
        n243 = Array Subset(array=w526, index=i32 ?, length=i32 ?) -> (w523:u8[])
        n244 = Array To Cluster(array=w526) -> (cluster=w558:T7)
        n245 = Unbundle By Name(w558) -> ("[16]"=w555:u8, "[17]"=w554:u8, "[18]"=w550:u8, "[19]"=w551:u8, "[20]"=w545:u8, "[21]"=w544:u8, "[22]"=w539:u8, "[23]"=w538:u8, "[24]"=w530:u8, "[25]"=w531:u8, "[26]"=w533:u8, "[27]"=w532:u8)
        n246 = Array Subset(array=w526, index=i32 ?, length=i32 ?) -> (w560:u8[])
        n247 = To Unsigned Word Integer(number=w554) -> (unsigned 16bit integer=w557:u16)
        n248 = To Unsigned Word Integer(number=w551) -> (unsigned 16bit integer=w553:u16)
        n249 = To Word Integer(number=w544) -> (16bit integer=w547:i16)
        n250 = To Unsigned Word Integer(number=w538) -> (unsigned 16bit integer=w542:u16)
        n251 = To Unsigned Word Integer(number=w531) -> (unsigned 16bit integer=w537:u16)
        n252 = To Unsigned Word Integer(number=w532) -> (unsigned 16bit integer=w535:u16)
        n253 = Byte Array To String(unsigned byte array=w560) -> (string=w559:string)
        n254 = Logical Shift(y=w529, x=w557) -> (x << y=w556:u16)
        n255 = Logical Shift(y=w529, x=w553) -> (x << y=w552:u16)
        n256 = Logical Shift(y=w529, x=w547) -> (x << y=w546:i16)
        n257 = Logical Shift(y=w529, x=w542) -> (x << y=w541:u16)
        n258 = Logical Shift(y=w529, x=w537) -> (x << y=w536:u16)
        n259 = Logical Shift(y=w529, x=w535) -> (x << y=w534:u16)
        n260 = Add(x=w555, y=w556) -> (x+y=w549:u16)
        n261 = Add(x=w550, y=w552) -> (x+y=w548:u16)
        n262 = Add(x=w545, y=w546) -> (x+y=w543:i16)
        n263 = Add(x=w539, y=w541) -> (x+y=w540:u16)
        n264 = Add(x=w530, y=w536) -> (x+y=w528:u16)
        n265 = Add(x=w533, y=w534) -> (x+y=w527:u16)
        n266 = for {
          N: i32 ? -> [_]
          tunnel: w523 -> [w582] mode=indexing
          shift-right: [w580] -> w521
          shift-left: string ? -> [w581]
          tunnel: w519 -> [w575]
          i -> [w578]
          n267 = case shown="1" w575 {
            tunnel: [string ? ("format string") string ? ("format string") string ? ("format string") string ? ("format string")] -> w579
            frame #0 {
            }
            frame #1 {
            }
            frame #2 {
            }
            frame #3 {
            }
          }
          n268 = To Byte Integer(number=w582) -> (8bit integer=w576:i8)
          n269 = Increment(x=w578) -> (x+1=w577:i32)
          n270 = Format Into String(format string=w579, initial string=w581, w577, w576) -> (resulting string=w580:string)  [unwired: 1 in, 1 out]
        }
        n271 = Format Into String(format string=w561, initial string=w565, w559, w549, w548, w543, w540, w528, w527, w521) -> (resulting string=w564:string)  [unwired: 1 in, 1 out]
      }
      n272 = Array Subset(array=w478, index=i32 ?, length=i32 ?) -> (w510:u8[])
      n273 = Array Subset(array=w478, index=i32 ?, length=i32 ?) -> (w505:u8[])
      n274 = Number To Boolean Array(number=w489) -> (Boolean array=w498:bool[])
      n275 = Greater Than 0?(x=w513) -> (x > 0?=w501:bool)
      n276 = Greater Than 0?(x=w511) -> (x > 0?=w503:bool)
      n277 = Byte Array To String(unsigned byte array=w510) -> (string=w509:string)
      n278 = Array To Cluster(array=w498) -> (cluster=w497:T2)
      n279 = case shown="True" w501 {
        tunnel: [string ? string ?] -> w500
        frame #0 {
        }
        frame #1 {
        }
      }
      n280 = call <vilib>:"Trim Whitespace.vi"("string"=w509) -> ("trimmed string"=w477:string)  [unwired: 1 in]
      n281 = Unbundle By Name(w497) -> ("Boolean array[0]"=w496:bool, "Boolean array[1]"=w495:bool, "Boolean array[2]"=w494:bool, "Boolean array[3]"=w493:bool)
      n282 = case shown="False" w503 {
        tunnel: [string ? string ?] -> w502
        frame #0 {
        }
        frame #1 {
        }
      }
      n283 = for {
        shift-right: [w595] -> w504
        shift-left: string ? -> [w596]
        tunnel: w505 -> [w597] mode=indexing
        i -> [w592]
        w593 = i32 ?
        n284 = Multiply(x=w593, y=w592) -> (x*y=w591:i32)
        n285 = for {
          N: w593 -> [_]
          shift-right: [w604] -> w594
          shift-left: string ? -> [w606]
          tunnel: w597 -> [w607]
          tunnel: w591 -> [w601]
          i -> [w602]
          n286 = Negate(x=w602) -> (-x=w608:i32)
          n287 = Add(x=w601, y=w602) -> (x+y=w600:i32)
          n288 = Logical Shift(y=w608, x=w607) -> (x << y=w609:u8)
          n289 = And(x=u8 ? ("width (-)"), y=w609) -> (x .and. y?=w599:u8)
          n290 = case shown="0, Default" w599 {
            tunnel: [string ? string ?] -> w603
            frame #0 {
            }
            frame #1 {
            }
          }
          n291 = Format Into String(format string=string ?, initial string=w606, w600, w603) -> (resulting string=w604:string)  [unwired: 1 in, 1 out]
        }
        n292 = Concatenate Strings(w596, w594) -> (w595:string)
      }
      n293 = Select(t=w491, s=w496, f=w492) -> (s? t:f=w488:string)
      n294 = Select(t=w491, s=w494, f=w492) -> (s? t:f=w486:string)
      n295 = Select(t=w491, s=w495, f=w492) -> (s? t:f=w487:string)
      n296 = Select(t=w491, s=w493, f=w492) -> (s? t:f=w485:string)
      n297 = Format Into String(format string=string ?, w479, w500, w502, w477, w504, w483, w488, w487, w486, w485, w482) -> (resulting string=w517:string)  [unwired: 2 in, 1 out]
    }
    frame #25 {
      # "SET_PROGRAM_DEFINITION"
    }
    frame #26 {
      # "GET_PROGRAM_CONSTANTS"
      n298 = Index Array(array=w615, index=i32 ?) -> (element=w619:u8)
      n299 = Index Array(array=w615, index=i32 ?) -> (element=w620:u8)
      n300 = To Unsigned Word Integer(number=w620) -> (unsigned 16bit integer=w623:u16)
      n301 = Logical Shift(y=i8 ?, x=w623) -> (x << y=w621:u16)
      n302 = for {
        N: i32 ? -> [_]
        shift-right: [w643] -> w614
        shift-left: string ? -> [w644]
        tunnel: w615 -> [w640]
        i -> [w638]
        w637 = i32 ? ("index")
        n303 = Multiply(x=w638, y=w637) -> (x*y=w639:i32)
        n304 = Add(x=w639, y=w637) -> (x+y=w636:i32)
        n305 = Array Subset(array=w640, index=w636, length=i32 ?) -> (w635:u8[])
        n306 = Array To Cluster(array=w635) -> (cluster=w634:cluster{"[0]":u8, "[1]":u8})
        n307 = Unbundle(w634) -> ("[0]"=w630:u8, "[1]"=w629:u8)
        n308 = To Unsigned Word Integer(number=w629) -> (unsigned 16bit integer=w633:u16)
        n309 = Logical Shift(y=i8 ?, x=w633) -> (x << y=w631:u16)
        n310 = Add(x=w630, y=w631) -> (x+y=w628:u16)
        n311 = Format Into String(format string=string ?, initial string=w644, w638, w628) -> (resulting string=w643:string)  [unwired: 1 in, 1 out]
      }
      n312 = Add(x=w619, y=w621) -> (x+y=w618:u16)
      n313 = Format Into String(format string=string ?, w618, w614) -> (resulting string=w626:string)  [unwired: 2 in, 1 out]
    }
    frame #27 {
      # "SET_PROGRAM_CONSTANTS"
    }
    frame #28 {
      w654 = string ?
      w655 = string ?
      # "Convert MS DateTime\nto LV DateTime"
      # "GET_CONFIGURABLE_DEVICE_PARAMETERS"
      n314 = Array To Cluster(array=w648) -> (cluster=w678:T8)
      n315 = Unbundle By Name(w678) -> ("DATA[0]"=w712:u8, "DATA[1]"=w710:u8, "DATA[2]"=w708:u8, "DATA[3]"=w707:u8, "DATA[4]"=w706:u8, "DATA[5]"=w703:u8, "DATA[6]"=w702:u8, "DATA[7]"=w701:u8, "DATA[8]"=w700:u8, "DATA[9]"=w697:u8, "DATA[10]"=w696:u8, "DATA[11]"=w695:u8)
      n316 = Unbundle By Name(w678) -> ("DATA[42]"=w675:u8, "DATA[43]"=w674:u8, "DATA[44]"=w671:u8, "DATA[45]"=w670:u8, "DATA[46]"=w659:u8)
      n317 = Index Array(array=w648, index=i32 ?) -> (element=w647:u8)
      n318 = Array Subset(array=w648, index=i32 ?, length=i32 ?) -> (w685:u8[])
      n319 = Array Subset(array=w648, index=i32 ?, length=i32 ?) -> (w680:u8[])
      n320 = for {
        tunnel: w685 -> [w722] mode=indexing
        shift-right: [w716] -> w690
        shift-left: u64 ? ("y") -> [w717]
        tunnel: i8 ? ("y") -> [w720]
        i -> [w721]
        n321 = To Unsigned Quad Integer(1:w722) -> (0:w715:u64)
        n322 = Multiply(x=w720, y=w721) -> (x*y=w719:i32)
        n323 = Logical Shift(y=w719, x=w715) -> (x << y=w718:u64)
        n324 = Add(x=w717, y=w718) -> (x+y=w716:u64)
      }
      n325 = Greater Than 0?(x=w712) -> (x > 0?=w711:bool)
      n326 = Greater Than 0?(x=w706) -> (x > 0?=w705:bool)
      n327 = Greater Than 0?(x=w700) -> (x > 0?=w699:bool)
      n328 = Byte Array To String(unsigned byte array=w680) -> (string=w679:string)
      n329 = To Unsigned Word Integer(number=w674) -> (unsigned 16bit integer=w677:u16)
      n330 = Number To Boolean Array(number=w670) -> (Boolean array=w668:bool[])
      n331 = Number To Boolean Array(number=w659) -> (Boolean array=w660:bool[])
      n332 = Logical Shift(y=i8 ?, x=w677) -> (x << y=w676:u16)
      n333 = Array To Cluster(array=w668) -> (cluster=w669:T2)
      n334 = Array To Cluster(array=w660) -> (cluster=w661:T2)
      n335 = Add(x=w675, y=w676) -> (x+y=w672:u16)
      n336 = Unbundle By Name(w669) -> ("Boolean array[0]"=w666:bool, "Boolean array[1]"=w667:bool, "Boolean array[2]"=w664:bool)
      n337 = Unbundle By Name(w661) -> ("Boolean array[0]"=w656:bool, "Boolean array[1]"=w658:bool, "Boolean array[2]"=w657:bool)
      n338 = Multiply(x=u64 ? ("y"), y=u64 ?) -> (x*y=w688:u64)
      n339 = Quotient & Remainder(x=w690, y=u64 ?) -> (floor(x/y)=w646:u64)  [unwired: 1 out]
      n340 = Subtract(x=w646, y=w688) -> (x-y=w686:u64)
      n341 = Format Date/Time String(seconds (now)=w686, UTC format=bool ?) -> (date/time string=w650:string)  [unwired: 1 in]
      n342 = Select(t=w655, s=w705, f=w654) -> (s? t:f=w704:string)
      n343 = Select(t=w655, s=w666, f=w654) -> (s? t:f=w665:string)
      n344 = Select(t=w655, s=w664, f=w654) -> (s? t:f=w662:string)
      n345 = Select(t=w655, s=w658, f=w654) -> (s? t:f=w652:string)
      n346 = Select(t=w655, s=w711, f=w654) -> (s? t:f=w709:string)
      n347 = Select(t=w655, s=w699, f=w654) -> (s? t:f=w698:string)
      n348 = Select(t=w655, s=w667, f=w654) -> (s? t:f=w663:string)
      n349 = Select(t=w655, s=w656, f=w654) -> (s? t:f=w653:string)
      n350 = Select(t=w655, s=w657, f=w654) -> (s? t:f=w651:string)
      n351 = Format Into String(format string=string ?, w709, w710, w708, w707, w704, w703, w702, w701, w698, w697, w696, w695, w679, w672, w671, w665, w663, w662, w653, w652, w651, w650, w647) -> (resulting string=w713:string)  [unwired: 2 in, 1 out]
    }
    frame #29 {
      # "SET_CONFIGURABLE_DEVICE_PARAMETERS"
    }
    frame #30 {
      w732 = string ?
      w731 = string ?
      w777 = i8 ? ("y")
      # "GET_PULSE_CONSTANTS"
      n352 = Array To Cluster(array=w798) -> (cluster=w799:T9)
      n353 = Unbundle By Name(w799) -> ("DATA[0]"=w776:u8, "DATA[1]"=w756:u8, "DATA[2]"=w775:u8, "DATA[3]"=w724:u8, "DATA[4]"=w774:u8, "DATA[5]"=w757:u8, "DATA[6]"=w773:u8, "DATA[7]"=w758:u8, "DATA[8]"=w772:u8, "DATA[9]"=w759:u8, "DATA[10]"=w771:u8, "DATA[11]"=w760:u8, "DATA[12]"=w770:u8, "DATA[13]"=w761:u8, "DATA[14]"=w769:u8, "DATA[15]"=w762:u8, "DATA[16]"=w768:u8, "DATA[17]"=w763:u8, "DATA[18]"=w767:u8, "DATA[19]"=w764:u8, "DATA[20]"=w766:u8, "DATA[21]"=w765:u8, "DATA[22]"=w730:u8, "DATA[23]"=w729:u8)
      n354 = To Unsigned Word Integer(number=w756) -> (unsigned 16bit integer=w801:u16)
      n355 = To Unsigned Word Integer(number=w724) -> (unsigned 16bit integer=w797:u16)
      n356 = To Unsigned Word Integer(number=w757) -> (unsigned 16bit integer=w795:u16)
      n357 = To Unsigned Word Integer(number=w758) -> (unsigned 16bit integer=w793:u16)
      n358 = To Unsigned Word Integer(number=w759) -> (unsigned 16bit integer=w791:u16)
      n359 = To Unsigned Word Integer(number=w760) -> (unsigned 16bit integer=w789:u16)
      n360 = To Unsigned Word Integer(number=w761) -> (unsigned 16bit integer=w787:u16)
      n361 = To Unsigned Word Integer(number=w762) -> (unsigned 16bit integer=w785:u16)
      n362 = To Unsigned Word Integer(number=w763) -> (unsigned 16bit integer=w783:u16)
      n363 = To Unsigned Word Integer(number=w764) -> (unsigned 16bit integer=w781:u16)
      n364 = To Unsigned Word Integer(number=w765) -> (unsigned 16bit integer=w779:u16)
      n365 = Logical Shift(y=w777, x=w801) -> (x << y=w800:u16)
      n366 = Logical Shift(y=w777, x=w797) -> (x << y=w796:u16)
      n367 = Logical Shift(y=w777, x=w795) -> (x << y=w794:u16)
      n368 = Logical Shift(y=w777, x=w793) -> (x << y=w792:u16)
      n369 = Logical Shift(y=w777, x=w791) -> (x << y=w790:u16)
      n370 = Logical Shift(y=w777, x=w789) -> (x << y=w788:u16)
      n371 = Logical Shift(y=w777, x=w787) -> (x << y=w786:u16)
      n372 = Logical Shift(y=w777, x=w785) -> (x << y=w784:u16)
      n373 = Logical Shift(y=w777, x=w783) -> (x << y=w782:u16)
      n374 = Logical Shift(y=w777, x=w781) -> (x << y=w780:u16)
      n375 = Logical Shift(y=w777, x=w779) -> (x << y=w778:u16)
      n376 = Add(x=w776, y=w800) -> (x+y=w755:u16)
      n377 = Add(x=w775, y=w796) -> (x+y=w754:u16)
      n378 = Add(x=w774, y=w794) -> (x+y=w753:u16)
      n379 = Add(x=w773, y=w792) -> (x+y=w752:u16)
      n380 = Add(x=w772, y=w790) -> (x+y=w751:u16)
      n381 = Add(x=w771, y=w788) -> (x+y=w750:u16)
      n382 = Add(x=w770, y=w786) -> (x+y=w749:u16)
      n383 = Add(x=w769, y=w784) -> (x+y=w748:u16)
      n384 = Add(x=w768, y=w782) -> (x+y=w747:u16)
      n385 = Add(x=w767, y=w780) -> (x+y=w746:u16)
      n386 = Add(x=w766, y=w778) -> (x+y=w733:u16)
      n387 = Number To Boolean Array(number=w746) -> (Boolean array=w745:bool[])
      n388 = Array To Cluster(array=w745) -> (cluster=w744:T10)
      n389 = Unbundle By Name(w744) -> ("Boolean array[0]"=w743:bool, "Boolean array[1]"=w742:bool, "Boolean array[2]"=w741:bool, "Boolean array[3]"=w736:bool, "Boolean array[4]"=w735:bool)
      n390 = Greater Than 0?(x=w730) -> (x > 0?=w728:bool)
      n391 = Greater Than 0?(x=w729) -> (x > 0?=w727:bool)
      n392 = Select(t=w731, s=w743, f=w732) -> (s? t:f=w740:string)
      n393 = Select(t=w731, s=w741, f=w732) -> (s? t:f=w738:string)
      n394 = Select(t=w731, s=w735, f=w732) -> (s? t:f=w734:string)
      n395 = Select(t=w731, s=w727, f=w732) -> (s? t:f=w725:string)
      n396 = Select(t=w731, s=w742, f=w732) -> (s? t:f=w739:string)
      n397 = Select(t=w731, s=w736, f=w732) -> (s? t:f=w737:string)
      n398 = Select(t=w731, s=w728, f=w732) -> (s? t:f=w726:string)
      n399 = Format Into String(format string=string ?, w755, w754, w753, w752, w751, w750, w749, w748, w747, w740, w739, w738, w737, w734, w733, w726, w725) -> (resulting string=w802:string)  [unwired: 2 in, 1 out]
    }
    frame #31 {
      # "SET_PULSE_CONSTANTS"
    }
    frame #32 {
      # "GET_LEAD_LIMITS"
      n400 = for {
        N: i32 ? -> [_]
        shift-right: [w850] -> w805
        shift-left: string ? -> [w851]
        tunnel: w807 -> [w847]
        i -> [w845]
        n401 = Multiply(x=w845, y=i32 ? ("index")) -> (x*y=w846:i32)
        n402 = Add(x=w846, y=i32 ?) -> (x+y=w843:i32)
        n403 = Array Subset(array=w847, index=w843, length=i32 ?) -> (w842:u8[])
        n404 = Increment(x=w845) -> (x+1=w833:i32)
        n405 = Array To Cluster(array=w842) -> (cluster=w841:cluster{"[0]":u8, "[1]":u8})
        n406 = Unbundle(w841) -> ("[0]"=w837:u8, "[1]"=w836:u8)
        n407 = To Unsigned Word Integer(number=w836) -> (unsigned 16bit integer=w840:u16)
        n408 = Logical Shift(y=i8 ?, x=w840) -> (x << y=w838:u16)
        n409 = Add(x=w837, y=w838) -> (x+y=w835:u16)
        n410 = Format Into String(format string=string ?, initial string=w851, w833, w835) -> (resulting string=w850:string)  [unwired: 1 in, 1 out]
      }
      n411 = for {
        N: i32 ? -> [_]
        shift-right: [w831] -> w806
        shift-left: string ? -> [w832]
        tunnel: w807 -> [w828]
        i -> [w826]
        n412 = Multiply(x=w826, y=i32 ? ("index")) -> (x*y=w827:i32)
        n413 = Add(x=w827, y=i32 ?) -> (x+y=w824:i32)
        n414 = Array Subset(array=w828, index=w824, length=i32 ?) -> (w823:u8[])
        n415 = Increment(x=w826) -> (x+1=w814:i32)
        n416 = Array To Cluster(array=w823) -> (cluster=w822:cluster{"[0]":u8, "[1]":u8})
        n417 = Unbundle(w822) -> ("[0]"=w818:u8, "[1]"=w817:u8)
        n418 = To Unsigned Word Integer(number=w817) -> (unsigned 16bit integer=w821:u16)
        n419 = Logical Shift(y=i8 ?, x=w821) -> (x << y=w819:u16)
        n420 = Add(x=w818, y=w819) -> (x+y=w816:u16)
        n421 = Format Into String(format string=string ?, initial string=w832, w814, w816) -> (resulting string=w831:string)  [unwired: 1 in, 1 out]
      }
      n422 = Format Into String(format string=string ?, w806, w805) -> (resulting string=w812:string)  [unwired: 2 in, 1 out]
    }
    frame #33 {
      # "SET_LEAD_LIMITS"
    }
    frame #34 {
      # "GET_CHANNEL_CALIBRATIONS"
      n423 = for {
        N: i32 ? -> [_]
        shift-right: [w898] -> w853
        shift-left: string ? -> [w899]
        tunnel: w855 -> [w895]
        i -> [w893]
        n424 = Multiply(x=w893, y=i32 ? ("index")) -> (x*y=w894:i32)
        n425 = Add(x=w894, y=i32 ?) -> (x+y=w891:i32)
        n426 = Array Subset(array=w895, index=w891, length=i32 ?) -> (w890:u8[])
        n427 = Increment(x=w893) -> (x+1=w881:i32)
        n428 = Array To Cluster(array=w890) -> (cluster=w889:cluster{"[0]":u8, "[1]":u8})
        n429 = Unbundle(w889) -> ("[0]"=w885:u8, "[1]"=w884:u8)
        n430 = To Unsigned Word Integer(number=w884) -> (unsigned 16bit integer=w888:u16)
        n431 = Logical Shift(y=i8 ?, x=w888) -> (x << y=w886:u16)
        n432 = Add(x=w885, y=w886) -> (x+y=w883:u16)
        n433 = Format Into String(format string=string ?, initial string=w899, w881, w883) -> (resulting string=w898:string)  [unwired: 1 in, 1 out]
      }
      n434 = for {
        N: i32 ? -> [_]
        shift-right: [w879] -> w854
        shift-left: string ? -> [w880]
        tunnel: w855 -> [w876]
        i -> [w874]
        n435 = Multiply(x=w874, y=i32 ? ("index")) -> (x*y=w875:i32)
        n436 = Add(x=w875, y=i32 ?) -> (x+y=w872:i32)
        n437 = Array Subset(array=w876, index=w872, length=i32 ?) -> (w871:u8[])
        n438 = Increment(x=w874) -> (x+1=w862:i32)
        n439 = Array To Cluster(array=w871) -> (cluster=w870:cluster{"[0]":u8, "[1]":u8})
        n440 = Unbundle(w870) -> ("[0]"=w866:u8, "[1]"=w865:u8)
        n441 = To Unsigned Word Integer(number=w865) -> (unsigned 16bit integer=w869:u16)
        n442 = Logical Shift(y=i8 ?, x=w869) -> (x << y=w867:u16)
        n443 = Add(x=w866, y=w867) -> (x+y=w864:u16)
        n444 = Format Into String(format string=string ?, initial string=w880, w862, w864) -> (resulting string=w879:string)  [unwired: 1 in, 1 out]
      }
      n445 = Format Into String(format string=string ?, w854, w853) -> (resulting string=w860:string)  [unwired: 2 in, 1 out]
    }
    frame #35 {
      # "SET_CHANNEL_CALIBRATIONS"
    }
    frame #36 {
      # "GET_STIM_ASIC_HV_CALIBRATIONS"
      n446 = for {
        N: i32 ? -> [_]
        shift-right: [w923] -> w901
        shift-left: string ? -> [w924]
        tunnel: w902 -> [w920]
        i -> [w918]
        n447 = Multiply(x=w918, y=i32 ? ("index")) -> (x*y=w919:i32)
        n448 = Add(x=w919, y=i32 ?) -> (x+y=w916:i32)
        n449 = Array Subset(array=w920, index=w916, length=i32 ?) -> (w915:u8[])
        n450 = Array To Cluster(array=w915) -> (cluster=w914:cluster{"[0]":u8, "[1]":u8})
        n451 = Unbundle(w914) -> ("[0]"=w910:u8, "[1]"=w909:u8)
        n452 = To Unsigned Word Integer(number=w909) -> (unsigned 16bit integer=w913:u16)
        n453 = Logical Shift(y=i8 ?, x=w913) -> (x << y=w911:u16)
        n454 = Add(x=w910, y=w911) -> (x+y=w908:u16)
        n455 = Format Into String(format string=string ?, initial string=w924, w918, w908) -> (resulting string=w923:string)  [unwired: 1 in, 1 out]
      }
      n456 = Format Into String(format string=string ?, w901) -> (resulting string=w905:string)  [unwired: 2 in, 1 out]
    }
    frame #37 {
      # "SET_STIM_ASIC_HV_CALIBRATIONS"
    }
    frame #38 {
      # "GET_CP_DATA"
      n457 = for {
        N: i32 ? -> [_]
        shift-right: [w936] -> w927
        shift-left: string ? -> [w937]
        tunnel: w928 -> [w933] mode=indexing
        tunnel: [w933] -> w926 mode=indexing
        i -> [w934]
        n458 = Format Into String(format string=string ?, initial string=w937, w934, w933) -> (resulting string=w936:string)  [unwired: 1 in, 1 out]
      }
      "CP_DATA" <- w926
      n459 = Format Into String(format string=string ?, w927) -> (resulting string=w931:string)  [unwired: 2 in, 1 out]
    }
    frame #39 {
      # "SET_CP_DATA"
    }
    frame #40 {
      # "OPEN_LOG"
      n460 = Array To Cluster(array=w954) -> (cluster=w955:T6)
      n461 = Unbundle By Name(w955) -> ("DATA[0]"=w953:u8, "DATA[5]"=w949:u8, "DATA[4]"=w948:u8, "DATA[3]"=w947:u8, "DATA[2]"=w946:u8, "DATA[9]"=w945:u8, "DATA[8]"=w944:u8, "DATA[7]"=w943:u8, "DATA[6]"=w942:u8)
      n462 = Join Numbers(hi=w949, lo=w948) -> ((hi.lo)=w952:u16)
      n463 = Join Numbers(hi=w947, lo=w946) -> ((hi.lo)=w951:u16)
      n464 = Join Numbers(hi=w945, lo=w944) -> ((hi.lo)=w950:u16)
      n465 = Join Numbers(hi=w943, lo=w942) -> ((hi.lo)=w939:u16)
      n466 = Join Numbers(hi=w952, lo=w951) -> ((hi.lo)=w941:u32)
      n467 = Join Numbers(hi=w950, lo=w939) -> ((hi.lo)=w940:u32)
      n468 = Format Into String(format string=string ?, w953, w941, w940) -> (resulting string=w956:string)  [unwired: 2 in, 1 out]
    }
    frame #41 {
      # "READ_LOG"
      n469 = Array To Cluster(array=w962) -> (cluster=w972:T6)
      n470 = Unbundle By Name(w972) -> ("DATA[0]"=w971:u8, "DATA[1]"=w963:u8, "DATA[5]"=w967:u8, "DATA[4]"=w966:u8, "DATA[3]"=w965:u8, "DATA[2]"=w964:u8)
      n471 = Join Numbers(hi=w967, lo=w966) -> ((hi.lo)=w969:u16)
      n472 = Join Numbers(hi=w965, lo=w964) -> ((hi.lo)=w970:u16)
      n473 = Join Numbers(hi=w969, lo=w970) -> ((hi.lo)=w968:u32)
      n474 = for {
        N: w963 -> [_]
        tunnel: w962 -> [w996]
        tunnel: i32 ? ("index") -> [w986]
        shift-right: [w990] -> w958
        shift-left: string ? -> [w989]
        tunnel: i32 ? ("index") -> [w987]
        i -> [w993]
        n475 = Multiply(x=w993, y=w986) -> (x*y=w994:i32)
        n476 = Add(x=w994, y=w987) -> (x+y=w995:i32)
        n477 = Array Subset(array=w996, index=w995, length=w986) -> (w992:u8[])
        n478 = Array To Cluster(array=w992) -> (cluster=w991:T11)
        n479 = Unbundle By Name(w991) -> ("[3]"=w983:u8, "[2]"=w982:u8, "[1]"=w981:u8, "[0]"=w980:u8, "[4]"=w978:u8, "[5]"=w977:u8, "[6]"=w976:u8, "[7]"=w975:u8)
        n480 = Join Numbers(hi=w983, lo=w982) -> ((hi.lo)=w984:u16)
        n481 = Join Numbers(hi=w981, lo=w980) -> ((hi.lo)=w985:u16)
        n482 = Join Numbers(hi=w984, lo=w985) -> ((hi.lo)=w979:u32)
        n483 = Format Into String(format string=string ?, initial string=w989, w979, w978, w977, w976, w975) -> (resulting string=w990:string)  [unwired: 1 in, 1 out]
      }
      n484 = Format Into String(format string=string ?, w971, w963, w968, w958) -> (resulting string=w973:string)  [unwired: 2 in, 1 out]
    }
    frame #42 {
      # "APPEND_LOG"
      n485 = Array To Cluster(array=w998) -> (cluster=w999:T6)
      n486 = disable-structure shown="Enabled" {
        disable-tunnel: w999 -> [w1009 w1011]
        disable-tunnel: [w1002 w1010] -> w997
        frame #0 {
          n487 = Unbundle By Name(w1009) -> ("DATA[3]"=w1008:u8, "DATA[2]"=w1007:u8, "DATA[1]"=w1006:u8, "DATA[0]"=w1005:u8)
          n488 = Join Numbers(hi=w1008, lo=w1007) -> ((hi.lo)=w1004:u16)
          n489 = Join Numbers(hi=w1006, lo=w1005) -> ((hi.lo)=w1003:u16)
          n490 = Join Numbers(hi=w1004, lo=w1003) -> ((hi.lo)=w1002:u32)
        }
        frame #1 {
          n491 = Unbundle By Name(w1011) -> ("DATA[0]"=w1010:u8)
        }
      }
      n492 = Format Into String(format string=string ?, w997) -> (resulting string=w1000:string)  [unwired: 2 in, 1 out]
    }
    frame #43 {
      # "GET_PATIENT_PROGRAM_RUN-TIME"
      n493 = Array To Cluster(array=w1020) -> (cluster=w1021:T6)
      n494 = Unbundle By Name(w1021) -> ("DATA[0]"=w1019:u8, "DATA[5]"=w1016:u8, "DATA[4]"=w1015:u8, "DATA[3]"=w1014:u8, "DATA[2]"=w1013:u8)
      n495 = Join Numbers(hi=w1016, lo=w1015) -> ((hi.lo)=w1018:u16)
      n496 = Join Numbers(hi=w1014, lo=w1013) -> ((hi.lo)=w1017:u16)
      n497 = Join Numbers(hi=w1018, lo=w1017) -> ((hi.lo)=w1012:u32)
      n498 = Format Into String(format string=string ?, w1019, w1012) -> (resulting string=w1022:string)  [unwired: 2 in, 1 out]
    }
    frame #44 {
      # "SET_PATIENT_PROGRAM_RUN-TIME"
    }
    frame #45 {
      # "IMPEDANCE_MEASUREMENT"
      n499 = Array To Cluster(array=w1028) -> (cluster=w1032:T6)
      n500 = Unbundle By Name(w1032) -> ("DATA[0]"=w1031:u8, "DATA[1]"=w1030:u8, "DATA[2]"=w1029:u8, "DATA[3]"=w1026:u8)
      n501 = for {
        N: w1026 -> [_]
        shift-right: [w1047] -> w1025
        shift-left: string ? -> [w1048]
        tunnel: w1028 -> [w1045]
        i -> [w1043]
        w1035 = i32 ? ("index")
        n502 = Multiply(x=w1043, y=w1035) -> (x*y=w1044:i32)
        n503 = Add(x=w1044, y=i32 ?) -> (x+y=w1042:i32)
        n504 = Array Subset(array=w1045, index=w1042, length=w1035) -> (w1041:u8[])
        n505 = Array To Cluster(array=w1041) -> (cluster=w1038:cluster{"[0]":u8, "[1]":u8})
        n506 = Unbundle By Name(w1038) -> ("[1]"=w1036:u8, "[0]"=w1037:u8)
        n507 = Join Numbers(hi=w1036, lo=w1037) -> ((hi.lo)=w1039:u16)
        n508 = Format Into String(format string=string ?, initial string=w1048, w1043, w1039) -> (resulting string=w1047:string)  [unwired: 1 in, 1 out]
      }
      n509 = Format Into String(format string=string ?, w1031, w1030, w1029, w1026, w1025) -> (resulting string=w1033:string)  [unwired: 2 in, 1 out]
    }
    frame #46 {
      # "ENTER_STORAGE_MODE"
    }
    frame #47 {
      # "Echo Short"
      n510 = Array Subset(array=w1053, index=i32 ?, length=i32 ?) -> (w1051:u8[])
      n511 = Byte Array To String(unsigned byte array=w1051) -> (string=w1050:string)
      n512 = Format Into String(format string=string ?, w1050) -> (resulting string=w1055:string)  [unwired: 2 in, 1 out]
    }
    frame #48 {
      # "Echo Long"
      n513 = Array Subset(array=w1058, index=i32 ?, length=i32 ?) -> (w1059:u8[])
      n514 = Byte Array To String(unsigned byte array=w1059) -> (string=w1057:string)
      n515 = Format Into String(format string=string ?, w1057) -> (resulting string=w1062:string)  [unwired: 2 in, 1 out]
    }
    frame #49 {
      # "GET_GENERAL_CALIBRATION"
      n516 = Array Subset(array=w1073, index=i32 ?, length=i32 ?) -> (w1092:u8[])
      n517 = Index Array(array=w1073, index=i32 ?) -> (element=w1097:u8)
      n518 = Index Array(array=w1073, index=i32 ?) -> (element=w1098:u8)
      n519 = Index Array(array=w1073, index=i32 ?) -> (element=w1094:u8)
      n520 = Index Array(array=w1073, index=i32 ?) -> (element=w1095:u8)
      n521 = Array Subset(array=w1073, index=i32 ?, length=i32 ?) -> (w1087:u8[])
      n522 = Array Subset(array=w1073, index=i32 ?, length=i32 ?) -> (w1084:u8[])
      n523 = Array Subset(array=w1073, index=i32 ?, length=i32 ?) -> (w1082:u8[])
      n524 = Index Array(array=w1073, index=i32 ?) -> (element=w1074:u8)
      n525 = Index Array(array=w1073, index=i32 ?) -> (element=w1075:u8)
      n526 = Join Numbers(hi=w1097, lo=w1098) -> ((hi.lo)=w1096:u16)
      n527 = Join Numbers(hi=w1094, lo=w1095) -> ((hi.lo)=w1093:u16)
      n528 = Join Numbers(hi=w1074, lo=w1075) -> ((hi.lo)=w1072:u16)
      n529 = for {
        N: i32 ? -> [_]
        shift-right: [w1160] -> w1090
        shift-left: string ? -> [w1161]
        tunnel: w1092 -> [w1158]
        i -> [w1156]
        w1148 = i32 ? ("index")
        n530 = Multiply(x=w1156, y=w1148) -> (x*y=w1157:i32)
        n531 = Add(x=w1157, y=i32 ?) -> (x+y=w1155:i32)
        n532 = Array Subset(array=w1158, index=w1155, length=w1148) -> (w1154:u8[])
        n533 = Array To Cluster(array=w1154) -> (cluster=w1151:cluster{"[0]":u8, "[1]":u8})
        n534 = Unbundle By Name(w1151) -> ("[1]"=w1149:u8, "[0]"=w1150:u8)
        n535 = Join Numbers(hi=w1149, lo=w1150) -> ((hi.lo)=w1152:u16)
        n536 = Format Into String(format string=string ?, initial string=w1161, w1156, w1152) -> (resulting string=w1160:string)  [unwired: 1 in, 1 out]
      }
      n537 = for {
        N: i32 ? -> [_]
        shift-right: [w1146] -> w1086
        shift-left: string ? -> [w1147]
        tunnel: w1087 -> [w1144]
        i -> [w1142]
        w1134 = i32 ? ("index")
        n538 = Multiply(x=w1142, y=w1134) -> (x*y=w1143:i32)
        n539 = Add(x=w1143, y=i32 ?) -> (x+y=w1141:i32)
        n540 = Array Subset(array=w1144, index=w1141, length=w1134) -> (w1140:u8[])
        n541 = Array To Cluster(array=w1140) -> (cluster=w1137:cluster{"[0]":u8, "[1]":u8})
        n542 = Unbundle By Name(w1137) -> ("[1]"=w1135:u8, "[0]"=w1136:u8)
        n543 = Join Numbers(hi=w1135, lo=w1136) -> ((hi.lo)=w1138:u16)
        n544 = Format Into String(format string=string ?, initial string=w1147, w1142, w1138) -> (resulting string=w1146:string)  [unwired: 1 in, 1 out]
      }
      n545 = for {
        N: i32 ? -> [_]
        shift-right: [w1132] -> w1079
        shift-left: string ? -> [w1133]
        tunnel: w1084 -> [w1130]
        i -> [w1128]
        w1120 = i32 ? ("index")
        n546 = Multiply(x=w1128, y=w1120) -> (x*y=w1129:i32)
        n547 = Add(x=w1129, y=i32 ?) -> (x+y=w1127:i32)
        n548 = Array Subset(array=w1130, index=w1127, length=w1120) -> (w1126:u8[])
        n549 = Array To Cluster(array=w1126) -> (cluster=w1123:cluster{"[0]":u8, "[1]":u8})
        n550 = Unbundle By Name(w1123) -> ("[1]"=w1121:u8, "[0]"=w1122:u8)
        n551 = Join Numbers(hi=w1121, lo=w1122) -> ((hi.lo)=w1124:u16)
        n552 = Format Into String(format string=string ?, initial string=w1133, w1128, w1124) -> (resulting string=w1132:string)  [unwired: 1 in, 1 out]
      }
      n553 = for {
        N: i32 ? -> [_]
        shift-right: [w1118] -> w1078
        shift-left: string ? -> [w1119]
        tunnel: w1082 -> [w1116]
        i -> [w1114]
        w1106 = i32 ? ("index")
        n554 = Multiply(x=w1114, y=w1106) -> (x*y=w1115:i32)
        n555 = Add(x=w1115, y=i32 ?) -> (x+y=w1113:i32)
        n556 = Array Subset(array=w1116, index=w1113, length=w1106) -> (w1112:u8[])
        n557 = Array To Cluster(array=w1112) -> (cluster=w1109:cluster{"[0]":u8, "[1]":u8})
        n558 = Unbundle By Name(w1109) -> ("[1]"=w1107:u8, "[0]"=w1108:u8)
        n559 = Join Numbers(hi=w1107, lo=w1108) -> ((hi.lo)=w1110:u16)
        n560 = Format Into String(format string=string ?, initial string=w1119, w1114, w1110) -> (resulting string=w1118:string)  [unwired: 1 in, 1 out]
      }
      n561 = Format Into String(format string=string ?, w1090, w1096, w1093, w1086, w1079, w1078, w1072) -> (resulting string=w1104:string)  [unwired: 2 in, 1 out]
    }
    frame #50 {
      # "SET_GENERAL_CALIBRATION"
    }
    frame #51 {
      # "GET_TRIM_LIST"
      n562 = Array To Cluster(array=w1166) -> (cluster=w1168:T6)
      n563 = Unbundle By Name(w1168) -> ("DATA[0]"=w1167:u8, "DATA[1]"=w1163:u8)
      n564 = for {
        N: w1163 -> [_]
        shift-right: [w1184] -> w1164
        shift-left: string ? -> [w1185]
        tunnel: w1166 -> [w1182]
        i -> [w1180]
        w1173 = i32 ? ("index")
        n565 = Multiply(x=w1180, y=w1173) -> (x*y=w1181:i32)
        n566 = Add(x=w1181, y=i32 ?) -> (x+y=w1179:i32)
        n567 = Array Subset(array=w1182, index=w1179, length=w1173) -> (w1178:u8[])
        n568 = Array To Cluster(array=w1178) -> (cluster=w1176:cluster{"[0]":u8, "[1]":u8, "[2]":u8})
        n569 = Unbundle By Name(w1176) -> ("[1]"=w1174:u8, "[0]"=w1175:u8, "[2]"=w1171:u8)
        n570 = Join Numbers(hi=w1174, lo=w1175) -> ((hi.lo)=w1172:u16)
        n571 = Format Into String(format string=string ?, initial string=w1185, w1172, w1171) -> (resulting string=w1184:string)  [unwired: 1 in, 1 out]
      }
      n572 = Format Into String(format string=string ?, w1167, w1163, w1164) -> (resulting string=w1169:string)  [unwired: 2 in, 1 out]
    }
    frame #52 {
      # "SET_TRIM_LIST"
    }
    frame #53 {
      # "GET_COUNTER"
      n573 = Array To Cluster(array=w1191) -> (cluster=w1190:T4)
      n574 = Unbundle By Name(w1190) -> ("DATA[0]"=w1189:u8, "DATA[2]"=w1188:u8, "DATA[3]"=w1187:u8)
      n575 = To Unsigned Word Integer(number=w1187) -> (unsigned 16bit integer=w1195:u16)
      n576 = Logical Shift(y=i8 ?, x=w1195) -> (x << y=w1193:u16)
      n577 = Add(x=w1188, y=w1193) -> (x+y=w1192:u16)
      n578 = Format Into String(format string=string ?, w1189, w1192) -> (resulting string=w1196:string)  [unwired: 2 in, 1 out]
    }
    frame #54 {
      # "SET_COUNTER"
    }
    frame #55 {
      # "GET_TEST_STIMULATION"
      n579 = Index Array(array=w1200, index #1=i32 ? ("index")) -> (element #1=w1203:u8, element #2=w1202:u8, element #3=w1201:u8)  [unwired: 2 in]
      n580 = for {
        N: i32 ? -> [_]
        shift-right: [w1240] -> w1199
        shift-left: string ? -> [w1241]
        tunnel: w1200 -> [w1230]
        i -> [w1231]
        w1210 = i32 ? ("index")
        w1245 = i32 ? ("length")
        n581 = Multiply(x=w1231, y=w1245) -> (x*y=w1243:i32)
        n582 = Add(x=i32 ? ("index"), y=w1243) -> (x+y=w1244:i32)
        n583 = Array Subset(array=w1230, index=w1244, length=w1245) -> (w1228:u8[])
        n584 = Array To Cluster(array=w1228) -> (cluster=w1223:T12)
        n585 = Array Subset(array=w1228, index=i32 ?, length=i32 ?) -> (w1234:u8[])
        n586 = Unbundle By Name(w1223) -> ("[31]"=w1222:u8, "[32]"=w1221:u8, "[33]"=w1220:u8, "[34]"=w1217:u8, "[35]"=w1216:u8, "[36]"=w1212:u8, "[37]"=w1211:u8)
        n587 = Unbundle By Name(w1223) -> ("[3]"=w1226:u8, "[4]"=w1227:u8)
        n588 = To Unsigned Word Integer(number=w1227) -> (unsigned 16bit integer=w1239:u16)
        n589 = for {
          N: i32 ? -> [_]
          tunnel: w1234 -> [w1246] mode=indexing
          shift-right: [w1252] -> w1224
          shift-left: string ? -> [w1253]
          tunnel: w1231 -> [w1247]
          i -> [w1250]
          n590 = case shown="3" w1247 {
            tunnel: [string ? ("format string") string ? ("format string") string ? ("format string") string ? ("format string")] -> w1251
            frame #0 {
            }
            frame #1 {
            }
            frame #2 {
            }
            frame #3 {
            }
          }
          n591 = To Byte Integer(number=w1246) -> (8bit integer=w1248:i8)
          n592 = Increment(x=w1250) -> (x+1=w1249:i32)
          n593 = Format Into String(format string=w1251, initial string=w1253, w1249, w1248) -> (resulting string=w1252:string)  [unwired: 1 in, 1 out]
        }
        n594 = To Unsigned Word Integer(number=w1216) -> (unsigned 16bit integer=w1218:u16)
        n595 = To Unsigned Word Integer(number=w1211) -> (unsigned 16bit integer=w1214:u16)
        n596 = Logical Shift(y=i32 ? ("index"), x=w1239) -> (x << y=w1238:u16)
        n597 = Logical Shift(y=w1210, x=w1218) -> (x << y=w1219:u16)
        n598 = Logical Shift(y=w1210, x=w1214) -> (x << y=w1213:u16)
        n599 = Add(x=w1226, y=w1238) -> (x+y=w1225:u16)
        n600 = Add(x=w1217, y=w1219) -> (x+y=w1215:u16)
        n601 = Add(x=w1212, y=w1213) -> (x+y=w1209:u16)
        n602 = Format Into String(format string=string ?, initial string=w1241, w1225, w1224, w1222, w1221, w1220, w1215, w1209) -> (resulting string=w1240:string)  [unwired: 1 in, 1 out]
      }
      n603 = Format Into String(format string=string ?, w1203, w1202, w1201, w1199) -> (resulting string=w1208:string)  [unwired: 2 in, 1 out]
    }
    frame #56 {
      # "SET_TEST_STIMULATION"
    }
    frame #57 {
      # "GET_TITRATION_STIMULATION"
      n604 = Index Array(array=w1260, index #1=i32 ? ("index")) -> (element #1=w1264:u8, element #2=w1263:u8)  [unwired: 1 in]
      n605 = for {
        N: i32 ? -> [_]
        shift-right: [w1290] -> w1259
        shift-left: string ? -> [w1291]
        tunnel: w1260 -> [w1281]
        i -> [w1282]
        w1270 = i32 ? ("index")
        w1295 = i32 ? ("length")
        n606 = Multiply(x=w1282, y=w1295) -> (x*y=w1293:i32)
        n607 = Add(x=i32 ? ("index"), y=w1293) -> (x+y=w1294:i32)
        n608 = Array Subset(array=w1281, index=w1294, length=w1295) -> (w1279:u8[])
        n609 = Array To Cluster(array=w1279) -> (cluster=w1275:T13)
        n610 = Array Subset(array=w1279, index=i32 ?, length=i32 ?) -> (w1285:u8[])
        n611 = Unbundle By Name(w1275) -> ("[2]"=w1277:u8, "[3]"=w1278:u8, "[4]"=w1272:u8, "[5]"=w1271:u8)
        n612 = To Unsigned Word Integer(number=w1278) -> (unsigned 16bit integer=w1289:u16)
        n613 = To Unsigned Word Integer(number=w1271) -> (unsigned 16bit integer=w1273:u16)
        n614 = for {
          N: i32 ? -> [_]
          tunnel: w1285 -> [w1296] mode=indexing
          shift-right: [w1302] -> w1268
          shift-left: string ? -> [w1303]
          tunnel: w1282 -> [w1297]
          i -> [w1300]
          n615 = case shown="3" w1297 {
            tunnel: [string ? ("format string") string ? ("format string") string ? ("format string") string ? ("format string")] -> w1301
            frame #0 {
            }
            frame #1 {
            }
            frame #2 {
            }
            frame #3 {
            }
          }
          n616 = To Byte Integer(number=w1296) -> (8bit integer=w1298:i8)
          n617 = Increment(x=w1300) -> (x+1=w1299:i32)
          n618 = Format Into String(format string=w1301, initial string=w1303, w1299, w1298) -> (resulting string=w1302:string)  [unwired: 1 in, 1 out]
        }
        n619 = Logical Shift(y=w1270, x=w1289) -> (x << y=w1288:u16)
        n620 = Logical Shift(y=w1270, x=w1273) -> (x << y=w1274:u16)
        n621 = Add(x=w1277, y=w1288) -> (x+y=w1276:u16)
        n622 = Add(x=w1272, y=w1274) -> (x+y=w1269:u16)
        n623 = Format Into String(format string=string ?, initial string=w1291, w1276, w1269, w1268) -> (resulting string=w1290:string)  [unwired: 1 in, 1 out]
      }
      n624 = Format Into String(format string=string ?, w1264, w1263, w1259) -> (resulting string=w1267:string)  [unwired: 2 in, 1 out]
    }
    frame #58 {
      # "SET_TITRATION_STIMULATION"
    }
    frame #59 {
      # "GET_RAMP_TIME"
      n625 = Array To Cluster(array=w1316) -> (cluster=w1315:cluster{"DATA[0]":u8, "DATA[1]":u8})
      n626 = Unbundle By Name(w1315) -> ("DATA[0]"=w1312:u8, "DATA[1]"=w1311:u8)
      n627 = To Unsigned Word Integer(number=w1311) -> (unsigned 16bit integer=w1310:u16)
      n628 = Logical Shift(y=i32 ? ("index"), x=w1310) -> (x << y=w1314:u16)
      n629 = Add(x=w1312, y=w1314) -> (x+y=w1309:u16)
      n630 = Format Into String(format string=string ?, w1309) -> (resulting string=w1317:string)  [unwired: 2 in, 1 out]
    }
    frame #60 {
      # "SET_RAMP_TIME"
    }
    frame #61 {
      # "GET_VBAT"
      n631 = Array To Cluster(array=w1321) -> (cluster=w1327:cluster{"DATA[0]":u8, "DATA[1]":u8})
      n632 = Unbundle By Name(w1327) -> ("DATA[0]"=w1324:u8, "DATA[1]"=w1323:u8)
      n633 = To Unsigned Word Integer(number=w1323) -> (unsigned 16bit integer=w1322:u16)
      n634 = Logical Shift(y=i32 ? ("index"), x=w1322) -> (x << y=w1326:u16)
      n635 = Add(x=w1324, y=w1326) -> (x+y=w1320:u16)
      n636 = Format Into String(format string=string ?, w1320) -> (resulting string=w1329:string)  [unwired: 2 in, 1 out]
    }
    frame #62 {
      (unwired) string ? ("format string")
      # "Not yet documented"
      # "SET_SOFTWARE_DESCRIPTION_BLOCK"
    }
    frame #63 {
      (unwired) string ? ("format string")
      # "Not yet documented"
      # "GET_SOFTWARE_DESCRIPTION_BLOCK"
    }
    frame #64 {
      # "WRITE_MEMORY"
    }
    frame #65 {
      # "READ_MEMORY"
      n637 = Array To Cluster(array=w1335) -> (cluster=w1351:T14)
      n638 = Unbundle By Name(w1351) -> ("DATA[3]"=w1348:u8, "DATA[2]"=w1347:u8, "DATA[1]"=w1346:u8, "DATA[0]"=w1345:u8, "DATA[4]"=w1337:u8, "DATA[5]"=w1338:u8)
      n639 = Array Subset(array=w1335, index=i32 ?, length=i32 ? ("index")) -> (w1332:u8[])
      n640 = Join Numbers(hi=w1348, lo=w1347) -> ((hi.lo)=w1350:u16)
      n641 = Join Numbers(hi=w1346, lo=w1345) -> ((hi.lo)=w1349:u16)
      n642 = Byte Array To String(unsigned byte array=w1332) -> (string=w1331:string)
      n643 = To Unsigned Word Integer(number=w1338) -> (unsigned 16bit integer=w1339:u16)
      n644 = Join Numbers(hi=w1350, lo=w1349) -> ((hi.lo)=w1342:u32)
      n645 = Logical Shift(y=i32 ? ("index"), x=w1339) -> (x << y=w1341:u16)
      n646 = Add(x=w1337, y=w1341) -> (x+y=w1336:u16)
      n647 = Format Into String(format string=string ?, w1342, w1336, w1331) -> (resulting string=w1343:string)  [unwired: 2 in, 1 out]
    }
    frame #66 {
      (unwired) string ? ("format string")
      # "Not yet documented"
      # "RESET_xPG"
    }
    frame #67 {
      (unwired) string ? ("format string")
      # "Not yet documented"
      # "ERASE_FLASH_BLOCK"
    }
    frame #68 {
      (unwired) string ? ("format string")
      # "Not yet documented"
      # "WRITE_VECTORS"
    }
    frame #69 {
      (unwired) string ? ("format string")
      # "Not yet documented"
      # "READ_VECTORS"
    }
    frame #70 {
      # "DIAGNOSTIC_DATA"
      n648 = Array To Cluster(array=w1363) -> (cluster=w1364:T14)
      n649 = Unbundle By Name(w1364) -> ("DATA[3]"=w1362:u8, "DATA[2]"=w1361:u8, "DATA[1]"=w1360:u8, "DATA[0]"=w1359:u8, "DATA[4]"=w1358:u8, "DATA[5]"=w1357:u8)
      n650 = Array Subset(array=w1363, index=i32 ?, length=i32 ?) -> (w1356:u8[])
      n651 = Join Numbers(hi=w1362, lo=w1361) -> ((hi.lo)=w1372:u16)
      n652 = Join Numbers(hi=w1360, lo=w1359) -> ((hi.lo)=w1371:u16)
      n653 = Byte Array To String(unsigned byte array=w1356) -> (string=w1352:string)
      n654 = To Unsigned Word Integer(number=w1357) -> (unsigned 16bit integer=w1368:u16)
      n655 = Logical Shift(y=i32 ? ("index"), x=w1368) -> (x << y=w1370:u16)
      n656 = Join Numbers(hi=w1372, lo=w1371) -> ((hi.lo)=w1354:u32)
      n657 = Add(x=w1358, y=w1370) -> (x+y=w1353:u16)
      n658 = Format Into String(format string=string ?, w1354, w1353, w1352) -> (resulting string=w1366:string)  [unwired: 2 in, 1 out]
    }
    frame #71 {
      # "SET_BACKGROUND_IMPEDANCE"
    }
    frame #72 {
      w1384 = i32 ? ("index")
      # "GET_BACKGROUND_IMPEDANCE"
      n659 = Array To Cluster(array=w1431) -> (cluster=w1430:T15)
      n660 = Unbundle By Name(w1430) -> ("DATA[0]"=w1427:u8, "DATA[1]"=w1426:u8, "DATA[2]"=w1422:u8, "DATA[3]"=w1421:u8, "DATA[4]"=w1417:u8, "DATA[5]"=w1416:u8, "DATA[6]"=w1412:u8, "DATA[7]"=w1411:u8, "DATA[8]"=w1401:u8, "DATA[9]"=w1400:u8, "DATA[10]"=w1396:u8, "DATA[11]"=w1395:u8, "DATA[12]"=w1385:u8, "DATA[13]"=w1391:u8, "DATA[14]"=w1386:u8, "DATA[15]"=w1387:u8, "DATA[16]"=w1375:u8)
      n661 = To Unsigned Word Integer(number=w1426) -> (unsigned 16bit integer=w1428:u16)
      n662 = To Unsigned Word Integer(number=w1421) -> (unsigned 16bit integer=w1424:u16)
      n663 = To Unsigned Word Integer(number=w1416) -> (unsigned 16bit integer=w1418:u16)
      n664 = To Unsigned Word Integer(number=w1411) -> (unsigned 16bit integer=w1414:u16)
      n665 = To Unsigned Word Integer(number=w1387) -> (unsigned 16bit integer=w1389:u16)
      n666 = To Unsigned Word Integer(number=w1391) -> (unsigned 16bit integer=w1392:u16)
      n667 = To Unsigned Word Integer(number=w1400) -> (unsigned 16bit integer=w1402:u16)
      n668 = To Unsigned Word Integer(number=w1395) -> (unsigned 16bit integer=w1398:u16)
      n669 = Greater Than 0?(x=w1375) -> (x > 0?=w1376:bool)
      n670 = Logical Shift(y=w1384, x=w1428) -> (x << y=w1429:u16)
      n671 = Logical Shift(y=w1384, x=w1424) -> (x << y=w1423:u16)
      n672 = Logical Shift(y=w1384, x=w1418) -> (x << y=w1419:u16)
      n673 = Logical Shift(y=w1384, x=w1414) -> (x << y=w1413:u16)
      n674 = Logical Shift(y=w1384, x=w1389) -> (x << y=w1388:u16)
      n675 = Logical Shift(y=w1384, x=w1392) -> (x << y=w1393:u16)
      n676 = Logical Shift(y=w1384, x=w1402) -> (x << y=w1403:u16)
      n677 = Logical Shift(y=w1384, x=w1398) -> (x << y=w1397:u16)
      n678 = case shown="True" w1376 {
        tunnel: [string ? string ?] -> w1374
        frame #0 {
        }
        frame #1 {
        }
      }
      n679 = Add(x=w1427, y=w1429) -> (x+y=w1425:u16)
      n680 = Add(x=w1422, y=w1423) -> (x+y=w1420:u16)
      n681 = Add(x=w1417, y=w1419) -> (x+y=w1415:u16)
      n682 = Add(x=w1412, y=w1413) -> (x+y=w1410:u16)
      n683 = Add(x=w1386, y=w1388) -> (x+y=w1382:u16)
      n684 = Add(x=w1385, y=w1393) -> (x+y=w1390:u16)
      n685 = Add(x=w1401, y=w1403) -> (x+y=w1399:u16)
      n686 = Add(x=w1396, y=w1397) -> (x+y=w1394:u16)
      n687 = Number To Boolean Array(number=w1410) -> (Boolean array=w1409:bool[])
      n688 = Number To Boolean Array(number=w1382) -> (Boolean array=w1383:bool[])
      n689 = Array To Cluster(array=w1409) -> (cluster=w1408:cluster{"Boolean array[0]":bool})
      n690 = Array To Cluster(array=w1383) -> (cluster=w1378:cluster{"Boolean array[0]":bool})
      n691 = Unbundle By Name(w1408) -> ("Boolean array[0]"=w1407:bool)
      n692 = Unbundle By Name(w1378) -> ("Boolean array[0]"=w1379:bool)
      n693 = Select(t=string ?, s=w1407, f=string ?) -> (s? t:f=w1404:string)
      n694 = Select(t=string ?, s=w1379, f=string ?) -> (s? t:f=w1377:string)
      n695 = Format Into String(format string=string ?, w1425, w1420, w1415, w1404, w1399, w1394, w1390, w1377, w1374) -> (resulting string=w1433:string)  [unwired: 2 in, 1 out]
    }
    frame #73 {
      # "Undefined"
    }
  }
  "Data" <- w18
  n696 = Unbundle By Name(w4) -> ("respToken"=w17:u8, "cmdToken"=w16:u16, "b1ChkSum"=w10:u8, "b1ChkSumCalc"=w9:u8, "tChkSum"=w8:u8, "tChkSumCalc"=w7:u8)
  n697 = case shown="43" w17 {
    selector: w17 -> [_ _ _ _ _ _ _ _ _ _ _ _ _ _ _ _ _ _ _ _ _ _ _ _ _ _ _ _ _ _ _ _ _ _ _ _ _ _ _ _ _ _ _ _ _ _ _ _ _ _ _ _ w1491 w1497 _]
    tunnel: [string ? string ? string ? string ? string ? string ? string ? string ? string ? string ? string ? string ? string ? string ? string ? string ? string ? string ? string ? string ? string ? string ? string ? string ? string ? string ? string ? string ? string ? string ? string ? string ? string ? string ? string ? string ? string ? string ? string ? string ? string ? string ? string ? string ? string ? string ? string ? string ? string ? string ? string ? string ? w1489 w1495 string ?] -> w23
    frame #0 {
    }
    frame #1 {
    }
    frame #2 {
    }
    frame #3 {
    }
    frame #4 {
    }
    frame #5 {
    }
    frame #6 {
    }
    frame #7 {
    }
    frame #8 {
    }
    frame #9 {
    }
    frame #10 {
    }
    frame #11 {
    }
    frame #12 {
    }
    frame #13 {
    }
    frame #14 {
    }
    frame #15 {
    }
    frame #16 {
    }
    frame #17 {
    }
    frame #18 {
    }
    frame #19 {
    }
    frame #20 {
    }
    frame #21 {
    }
    frame #22 {
    }
    frame #23 {
    }
    frame #24 {
    }
    frame #25 {
    }
    frame #26 {
    }
    frame #27 {
    }
    frame #28 {
    }
    frame #29 {
    }
    frame #30 {
    }
    frame #31 {
    }
    frame #32 {
    }
    frame #33 {
    }
    frame #34 {
    }
    frame #35 {
    }
    frame #36 {
    }
    frame #37 {
    }
    frame #38 {
    }
    frame #39 {
    }
    frame #40 {
    }
    frame #41 {
    }
    frame #42 {
    }
    frame #43 {
    }
    frame #44 {
    }
    frame #45 {
    }
    frame #46 {
    }
    frame #47 {
    }
    frame #48 {
    }
    frame #49 {
    }
    frame #50 {
    }
    frame #51 {
    }
    frame #52 {
      n698 = Number To Hexadecimal String(1:i16 ? ("width (-)"), 2:w1491) -> (0:w1490:string)
      n699 = Concatenate Strings(string ?, w1490, string ?) -> (w1489:string)
    }
    frame #53 {
      n700 = Number To Hexadecimal String(1:i16 ? ("width (-)"), 2:w1497) -> (0:w1496:string)
      n701 = Concatenate Strings(string ?, w1496, string ?) -> (w1495:string)
    }
    frame #54 {
    }
  }
  "Response Code" <- w23
  n702 = Equal?(x=w10, y=w9) -> (x = y?=→"bChecksum Valid":bool)
  n703 = Equal?(x=w8, y=w7) -> (x = y?=→"tChecksum Valid":bool)
  n704 = case shown="25" w16 {
    tunnel: [string ? string ? string ? string ? string ? string ? string ? string ? string ? string ? string ? string ? string ? string ? string ? string ? string ? string ? string ? string ? string ? string ? string ? string ? string ? string ? string ? string ? string ? string ? string ? string ? string ? string ? string ? string ? string ? string ? string ? string ? string ? string ? string ? string ? string ? string ? string ? string ? string ? string ? string ? string ? string ? string ? string ? string ? string ? string ? string ? string ? string ? string ? string ? string ?] -> w24
    frame #0 {
    }
    frame #1 {
    }
    frame #2 {
    }
    frame #3 {
    }
    frame #4 {
    }
    frame #5 {
    }
    frame #6 {
    }
    frame #7 {
    }
    frame #8 {
    }
    frame #9 {
    }
    frame #10 {
    }
    frame #11 {
    }
    frame #12 {
    }
    frame #13 {
    }
    frame #14 {
    }
    frame #15 {
    }
    frame #16 {
    }
    frame #17 {
    }
    frame #18 {
    }
    frame #19 {
    }
    frame #20 {
    }
    frame #21 {
    }
    frame #22 {
    }
    frame #23 {
    }
    frame #24 {
    }
    frame #25 {
    }
    frame #26 {
    }
    frame #27 {
    }
    frame #28 {
    }
    frame #29 {
    }
    frame #30 {
    }
    frame #31 {
    }
    frame #32 {
    }
    frame #33 {
    }
    frame #34 {
    }
    frame #35 {
    }
    frame #36 {
    }
    frame #37 {
    }
    frame #38 {
    }
    frame #39 {
    }
    frame #40 {
    }
    frame #41 {
    }
    frame #42 {
    }
    frame #43 {
    }
    frame #44 {
    }
    frame #45 {
    }
    frame #46 {
    }
    frame #47 {
    }
    frame #48 {
    }
    frame #49 {
    }
    frame #50 {
    }
    frame #51 {
    }
    frame #52 {
    }
    frame #53 {
    }
    frame #54 {
    }
    frame #55 {
    }
    frame #56 {
    }
    frame #57 {
    }
    frame #58 {
    }
    frame #59 {
    }
    frame #60 {
    }
    frame #61 {
    }
    frame #62 {
    }
    frame #63 {
    }
  }
  "Response Token" <- w24
  "error out" <- "error in (no error)"
